vi "GeneralPurposeSOS.vi"() -> ()   [LabVIEW 2015]
uses:
  <userlib>/atmcd32d.llb/EMGainMode_mode typedef.ctl
  <userlib>/atmcd32d.llb/ReadMode_mode typedef.ctl
  <userlib>/atmcd32d.llb/TriggerMode_mode typedef.ctl
  <userlib>/atmcd32d.llb/AcquisitionMode_mode typedef.ctl
  <userlib>/atmcd32d.llb/Shutter_type typedef.ctl
  <userlib>/atmcd32d.llb/Shutter_mode typedef.ctl
  <userlib>/atmcd32d.llb/Spool_method typedef.ctl
  <userlib>/atmcd32d.llb/Tiff_type typedef.ctl
  <vilib>/vision/NI_Vision_Development_Module.lvlib
  <userlib>/libtiff3.llb/libtiff3.lvlib
panel:
  in  "Cooling On":bool
  out "Current Frame 2":i32
  out "Cooling 2":bool
  out "Current T(°C) 2":i32
  in  "Camera Selection":T1(tab)
  in  "Exposure Time(s)":sgl min=0 step=0.1 format="%.2f"
  in  "Camera T(°C)":i32 min=-80 step=1
  in  "Camera DAQ Mode":T2(ring)=enum."Kinetics Series Scan"
  in  "Number of Frames to Acquire":i32 min=0 step=1
  in  "Exposure Time(s) 2":sgl min=0 step=0.1 format="%.2f"
  in  "Camera T(°C)  2":i32 min=-60 step=1
  in  "Camera DAQ Mode 2":T2(ring)=enum."Kinetics Series Scan"
  in  "Number of Frames to Acquire 2":i32 min=0 step=1
  in  "Illumination Mode":enum16{"TIRF", "Dark-Field"}(ring)
  in  "Flip Mirror 2":refnum<k7>(container)
  in  "Save Button":bool
  out "Camera On 2":bool
  out "Current Traj#":u32
  in  "Quit Program":bool
  out "Current Frame":i32
  in  "Start":bool
  in  "Stop":bool
  out "Cooling":bool
  out "Ready":bool
  out "Spot Index":i32
  out "Spot Center":cluster{"X":sgl, "Y":sgl}
  in  "Trajectory Length (s)":dbl=5.0 min=0.0 step=1.0 format="%#_13g"
  in  "Spot Choosing Region":enum16{"Donor", "Acceptor", "Entire Image"}(ring)
  in  "Flip Mirror 1":refnum<k7>(container)
  out "Image View":T3(tab)
  out "Image 3":T4(plugin-control)
  out "Image":T4(plugin-control)
  out "Trajectory":cluster{i32, i32}(graph)
  in  "Terminate Trajectory":bool
  out "error out":errorcluster
  out "Image 2":T4(plugin-control)
  in  "Number of Traj to Acquire":u32 step=1
  in  "Detection Mode":T5(ring)
  in  "Data Saving Path":path
  in  "Experiment Name":string
  out "Camera On":bool
  in  "System Shut Down":bool
  out "Current T(°C)":i32
  # "General-Purpose Single-Object Spectroscopy"
  # "System Settings"
  # "Wide-Field Camera Status"
  # "Spectrograph Status"
  # "Camera Settings"
  # "TIRF-Confocal Settings"
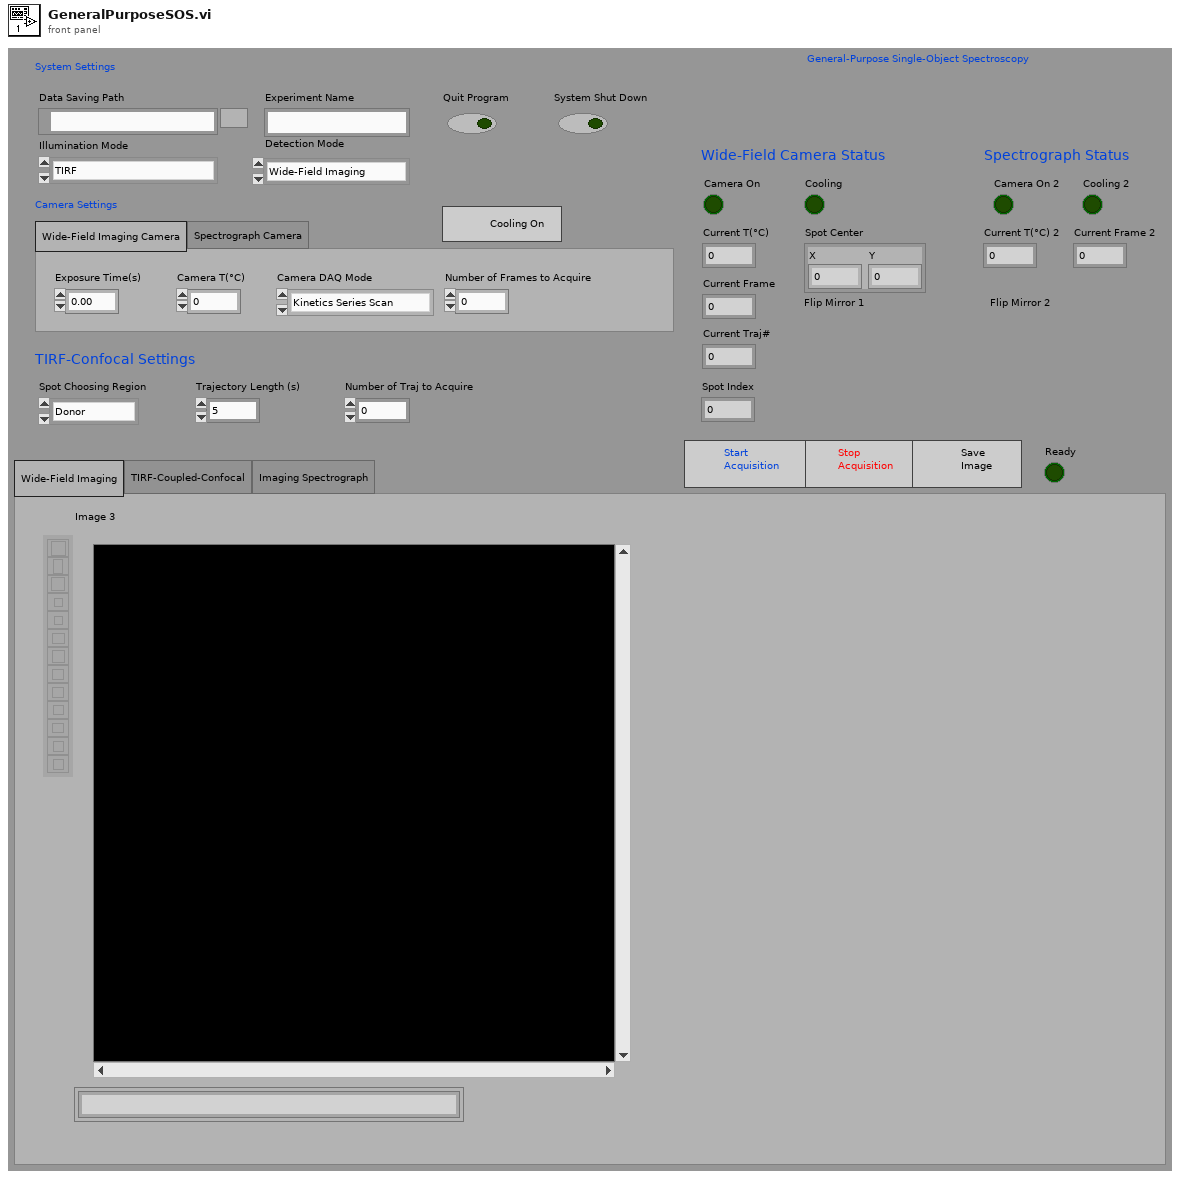
[diagram p1: front panel]
types:
  T1 = enum32{"Wide-Field Imaging Camera", "Spectrograph Camera"}
  T2 = enum16{"Live Monitoring", "Kinetics Series Scan"}
  T3 = enum32{"Wide-Field Imaging", "TIRF-Coupled-Confocal", "Imaging Spectrograph"}
  T4 = typedef "IMAQ Image.ctl" = refnum<image>
  T5 = enum16{"Wide-Field Imaging", "TIRF-Coupled-Confocal", "Imaging Spectrograph"}
  T6 = typedef "AcquisitionMode_mode typedef.ctl" = enum16{"Reserved (0)", "Single Scan", "Accumulate", "Kinetics", "Fast Kinetics", "Run Till Abort", "Reserved (6)", "Reserved (7)", "Reserved (8)", "Time Delayed Integration"}
  T7 = typedef "TriggerMode_mode typedef.ctl" = enum16{"Internal", "External", "N/A (2)", "N/A (3)", "N/A (4)", "N/A (5)", "External Start", "External Exposure (Bulb)", "N/A (8)", "External FVB EM", "Software", "N/A (11)", "External Charge Shifting"}
  T8 = typedef "ReadMode_mode typedef.ctl" = enum16{"Full Vertical Binning", "Multi-Track", "Random-Track", "Single-Track", "Image"}
  T9 = typedef "EMGainMode_mode typedef.ctl" = enum16{"8-bit", "12-bit", "Linear", "Real"}
  T10 = typedef "Shutter_mode typedef.ctl" = enum16{"Auto", "Open", "Close", "N/A (3)", "Open FVB Series", "Open Any Series"}
  T11 = typedef "Shutter_type typedef.ctl" = enum16{"TTL Low", "TTL High"}
  T12 = enum8{"Enabled", "Disabled", "Disabled and Grayed Out"}
  T13 = typedef "Spool_method typedef.ctl" = enum16{"32-bit", "Depends", "16-bit", "Multiple Directory", "Spool to RAM disk", "16-bit FITS", "SIF", "16-buit TIFF", "Multiple Directory Compressed"}
  T14 = typedef "IMAQ Rectangle" = cluster{"Left":i32, "Top":i32, "Right":i32, "Bottom":i32, "Rotation":dbl}
  T15 = typedef "Tiff_type typedef.ctl" = enum16{"8-bit", "16-bit", "color"}
  T16 = typedef "Error Code Enum typedef.ctl" = enum32{"N/A (0)", "DRV_ERROR_CODES", "DRV_SUCCESS", "DRV_VXDNOTINSTALLED", "DRV_ERROR_SCAN", "DRV_ERROR_CHECK_SUM", "DRV_ERROR_FILELOAD", "DRV_UNKNOWN_FUNC", "DRV_ERROR_VXD_INIT", "DRV_ERROR_ADDRESS", "DRV_ERROR_PAGELOCK", "DRV_ERROR_PAGEUNLOCK", "DRV_ERROR_BOARDTEST", "DRV_ERROR_ACK", "DRV_ERROR_UP_FIFO", "DRV_ERROR_PATTERN", "N/A (16)", "DRV_ACQUISITION_ERRORS", "DRV_ACQ_BUFFER", "DRV_ACQ_DOWNFIFO_FULL", "DRV_PROC_UNKONWN_INSTRUCTION", "DRV_ILLEGAL_OP_CODE", "DRV_KINETIC_TIME_NOT_MET", "DRV_ACCUM_TIME_NOT_MET", "DRV_NO_NEW_DATA", "N/A (25)", "DRV_SPOOLERROR", "N/A (27)", "N/A (28)", "N/A (29)", "N/A (30)", "N/A (31)", "N/A (32)", "DRV_TEMPERATURE_CODES", "DRV_TEMPERATURE_OFF", "DRV_TEMPERATURE_NOT_STABILIZED", "DRV_TEMPERATURE_STABILIZED", "DRV_TEMPERATURE_NOT_REACHED", "DRV_TEMPERATURE_OUT_RANGE", "DRV_TEMPERATURE_NOT_SUPPORTED", "DRV_TEMPERATURE_DRIFT", "N/A (41)", "N/A (42)", "N/A (43)", "N/A (44)", "N/A (45)", "N/A (46)", "N/A (47)", "N/A (48)", "DRV_GENERAL_ERRORS", "DRV_INVALID_AUX", "DRV_COF_NOTLOADED", "DRV_FPGAPROG", "DRV_FLEXERROR", "DRV_GPIBERROR", "N/A (55)", "N/A (56)", "N/A (57)", "N/A (58)", "N/A (59)", "N/A (60)", "N/A (61)", "N/A (62)", "N/A (63)", "DRV_DATATYPE", "DRV_DRIVER_ERRORS", "DRV_P1INVALID", "DRV_P2INVALID", "DRV_P3INVALID", "DRV_P4INVALID", "DRV_INIERROR", "DRV_COFERROR", "DRV_ACQUIRING", "DRV_IDLE", "DRV_TEMPCYCLE", "DRV_NOT_INITIALIZED", "DRV_P5INVALID", "DRV_P6INVALID", "DRV_INVALID_MODE", "DRV_INVALID_FILTER", "DRV_I2CERRORS", "DRV_I2CDEVNOTFOUND", "DRV_I2CTIMEOUT", "DRV_P7INVALID", "N/A (84)", "N/A (85)", "N/A (86)", "N/A (87)", "N/A (88)", "N/A (89)", "DRV_IOCERROR", "DRV_VRMVERSIONERROR"}
  T17 = typedef "Image Type" = u32
  T18 = cluster{"Objects":u16, "Threshold":i32, "Reject Border":bool, "Fill Holes":bool, "Min Object Size":bool, "Min Size":i32, "Max Object Size":bool, "Max Size":i32, "Show Search Area":bool, "Show Center":bool, "Show Bounding Box":bool}
  T19 = cluster{"Mean Intensity":sgl, "Standard  Deviation":sgl, "Minimum Intensity":sgl, "Maximum Intensity":sgl}
  T20 = cluster{"Object Center":cluster{"X":sgl, "Y":sgl}, "Bounding Box":cluster{"X Left":i32, "Y Top":i32, "X Right":i32, "Y Bottom":i32}, "Area":sgl, "Orientation":sgl, "Aspect Ratio":sgl, "Nb Holes":i32}[]
  T21 = cluster{"Nb pts X":u32, "Nb pts Y":u32, "xmin":dbl, "xmax":dbl, "ymin":dbl, "ymax":dbl}
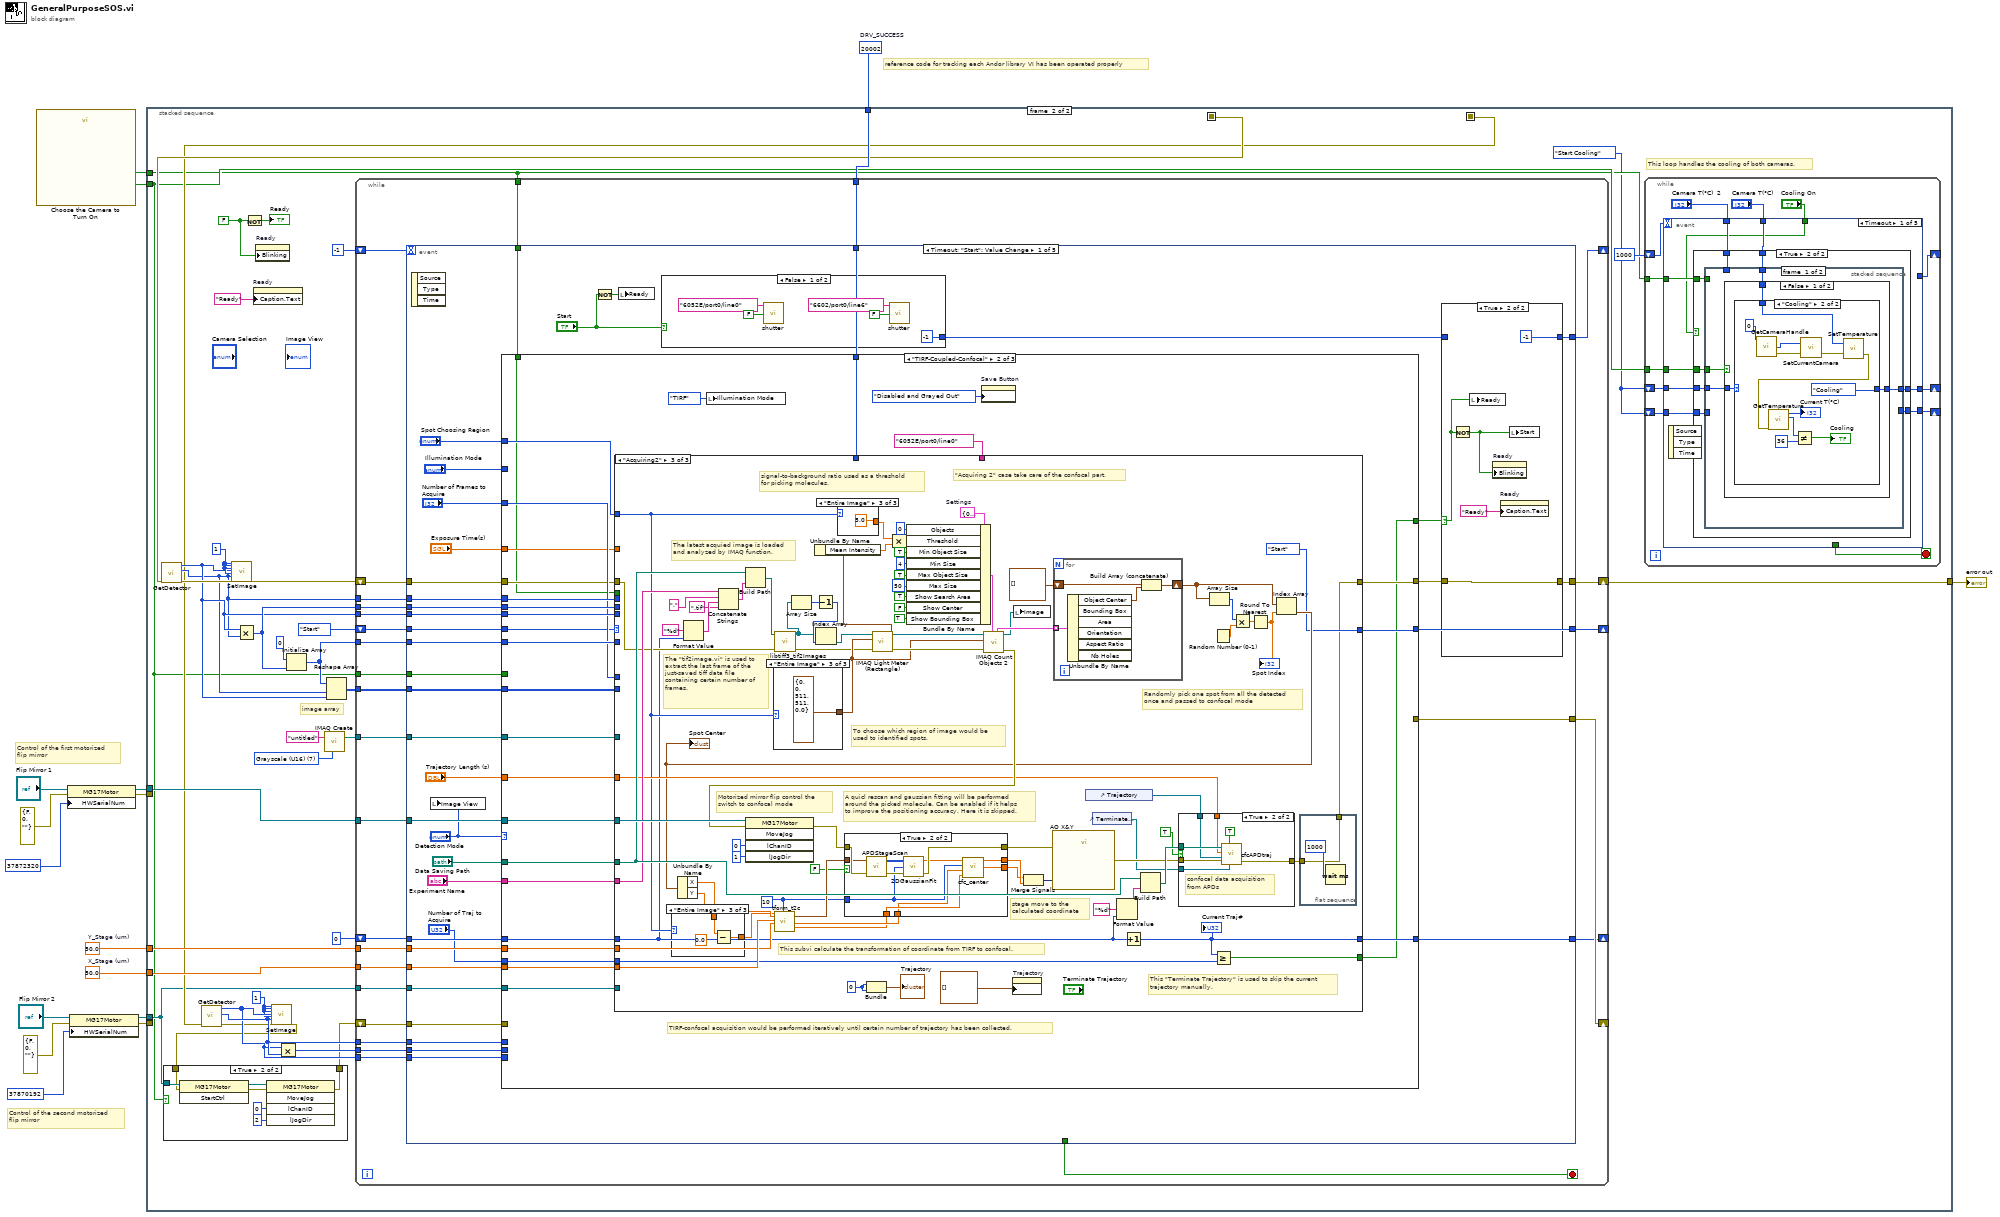
[diagram p0: block diagram]
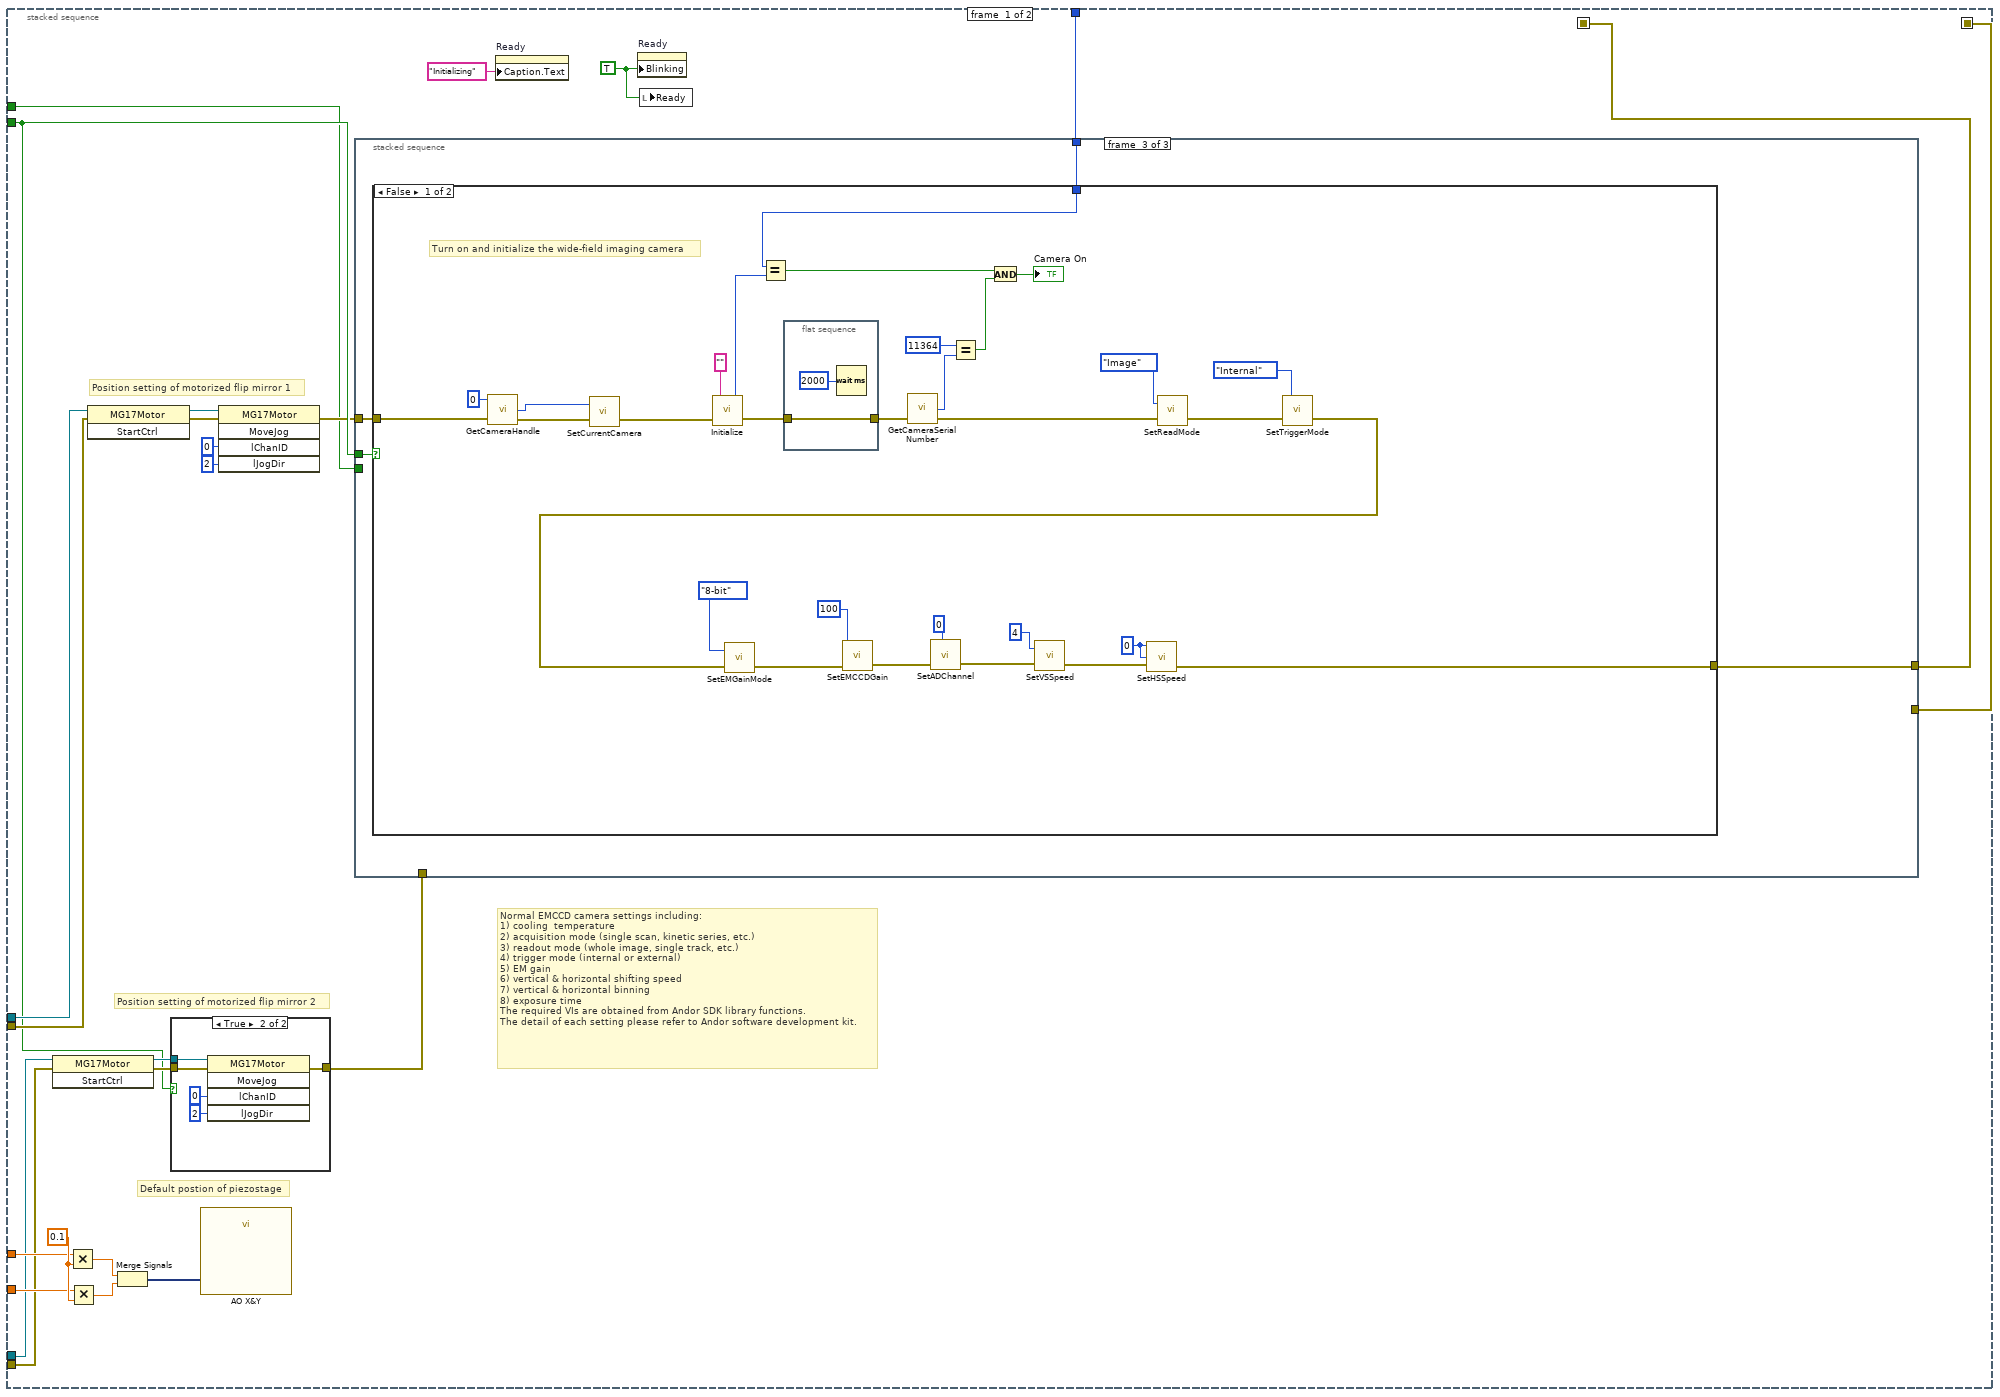
[diagram p2: hidden frame]
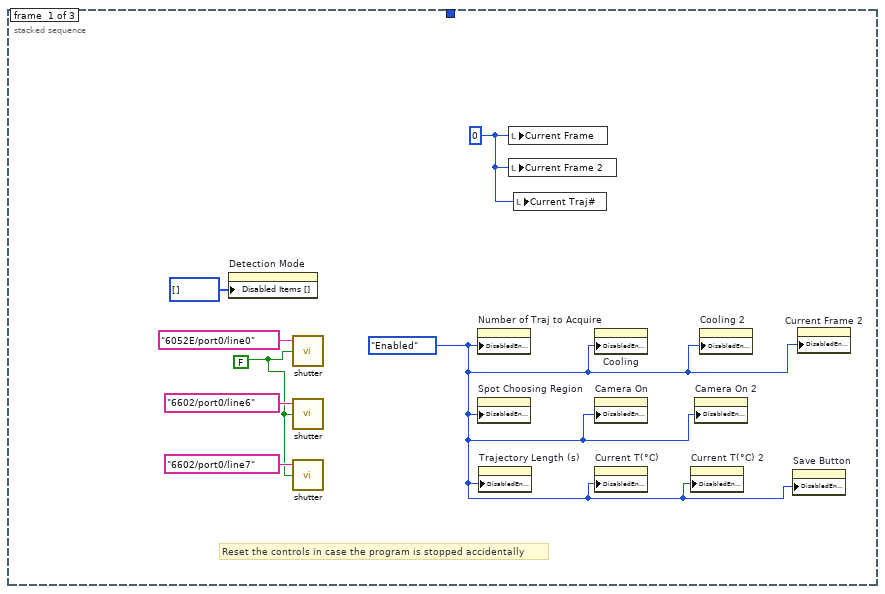
[diagram p3: hidden frame]
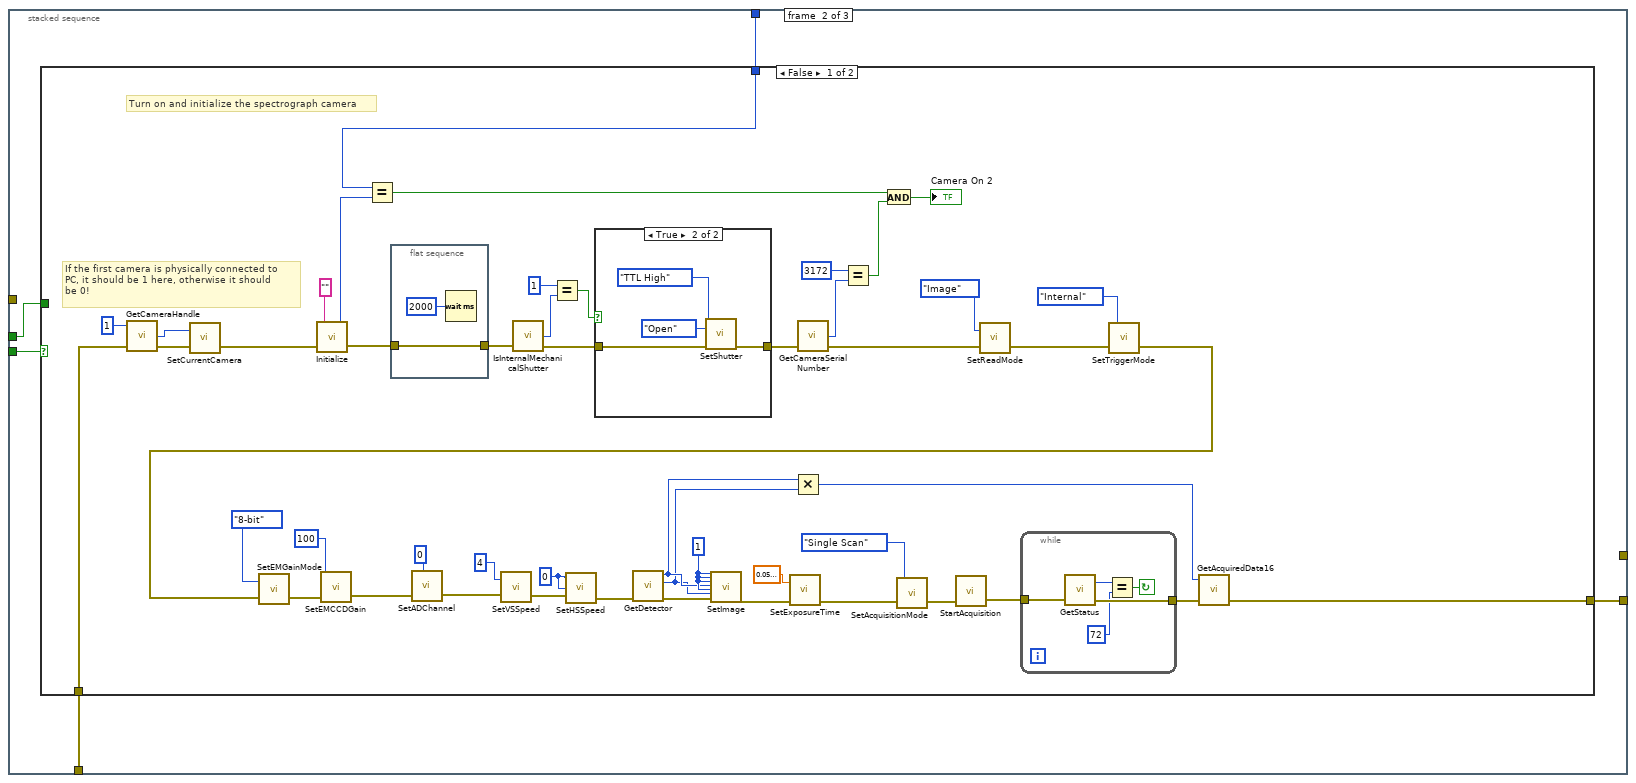
[diagram p4: hidden frame]
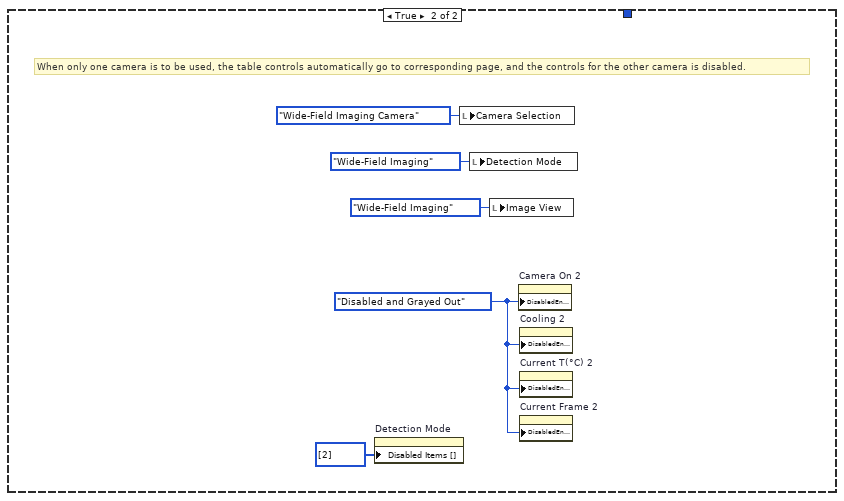
[diagram p6: hidden frame]
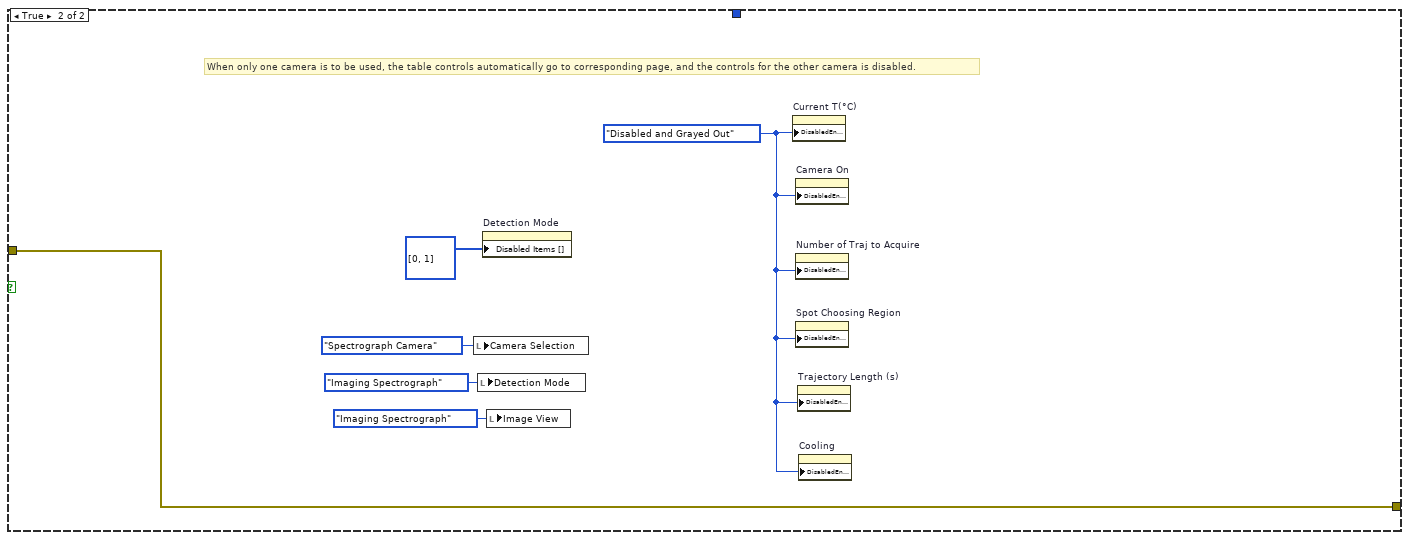
[diagram p7: hidden frame]
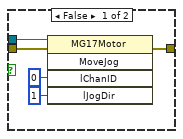
[diagram p8: hidden frame]
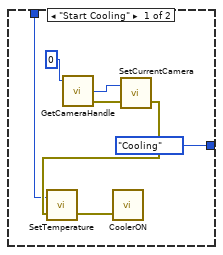
[diagram p10: hidden frame]
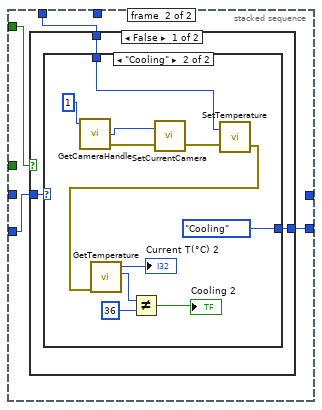
[diagram p12: hidden frame]
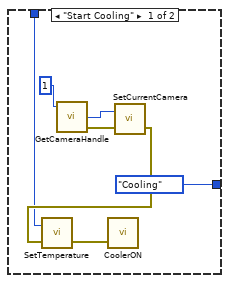
[diagram p13: hidden frame]
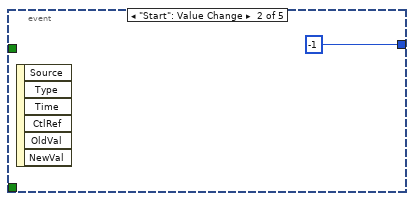
[diagram p15: hidden frame]
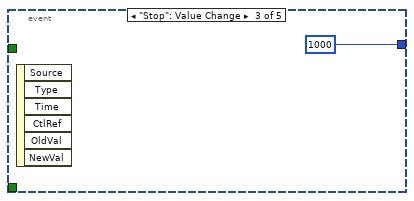
[diagram p16: hidden frame]
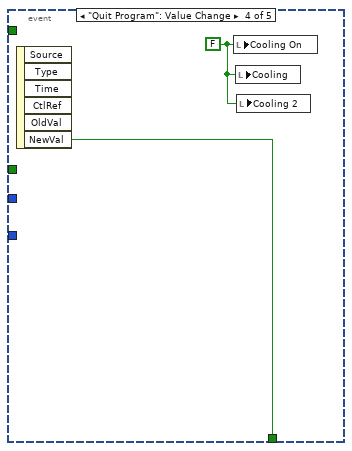
[diagram p17: hidden frame]
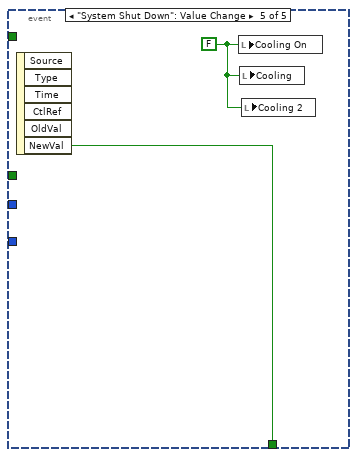
[diagram p18: hidden frame]
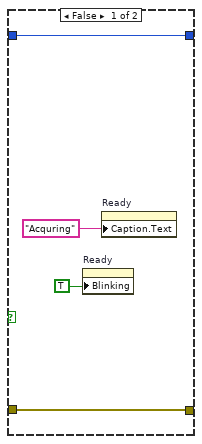
[diagram p20: hidden frame]
diagram:
  w9 = 50.0  # X_Stage (um)
  w10 = 50.0  # Y_Stage (um)
  w16 = 20002  # DRV_SUCCESS
  # "Control of the second motorized \nflip mirror"
  # "Control of the first motorized \nflip mirror"
  # "reference code for tracking each Andor library VI has been operated properly"
  n1 = call "Choose the Camera to Turn On"() -> ("Use spectrograpah camera"=w6:bool, "User wide-field camera"=w7:bool)  [unwired: 16 in, 2 out]
  n2 = property class="MG17Motor"(reference="Flip Mirror 1", error in=errorcluster {"status"=FALSE, "code"=0, "source"=""} ("error in (no error)"), "HWSerialNum"=37872320) -> (reference out=w12:refnum<k7>, error out=w11:errorcluster)
  n3 = property class="MG17Motor"(reference="Flip Mirror 2", error in=errorcluster {"status"=FALSE, "code"=0, "source"=""} ("error in (no error)"), "HWSerialNum"=37870192) -> (reference out=w2:refnum<k7>, error out=w1:errorcluster)
  n4 = stacked-sequence {
    seq-local: [w28 _] -> [_ w189]
    seq-local: [w19 _] -> [_ w185]
    tunnel: w16 -> [w41 w196]
    tunnel: w12 -> [w36 w199]
    tunnel: w11 -> [w35 _]
    tunnel: w10 -> [w32 w197]
    tunnel: w9 -> [w31 w198]
    tunnel: [_ w194] -> w8
    tunnel: w7 -> [w21 w176]
    tunnel: w6 -> [w23 w177]
    tunnel: w2 -> [w25 w182]
    tunnel: w1 -> [w24 _]
    frame #0 {
      w17 = TRUE ("Blinking")
      w33 = 0.1
      # "Position setting of motorized flip mirror 2"
      # "Normal EMCCD camera settings including:\n1) cooling  temperature\n2) acquisition mode (single scan, kinetic series, etc.)\n3) readout mode (whole image, single track, etc.)\n4) trigger mode (internal or external)\n5) EM gain \n6) vertical & horizontal shifting speed\n7) vertical & horizontal binning\n8) exposure time\nThe required VIs are obtained from Andor SDK library functions. \nThe detail of each setting please refer to Andor software development kit."
      # "Position setting of motorized flip mirror 1"
      # "Default postion of piezostage"
      n5 = invoke class="MG17Motor" method="StartCtrl"(reference=w25, error in=w24) -> (reference out=w27:refnum<k7>, error out=w26:errorcluster)  [unwired: 1 in, 1 out]
      n6 = Multiply(x=w32, y=w33) -> (x*y=w30:dbl)
      n7 = Multiply(x=w31, y=w33) -> (x*y=w29:dbl)
      n8 = invoke class="MG17Motor" method="StartCtrl"(reference=w36, error in=w35) -> (reference out=w40:refnum<k7>, error out=w39:errorcluster)  [unwired: 1 in, 1 out]
      n9 = Merge Signals(w30, w29) -> (w34:dynamicdata)
      n10 = case shown="True" w23 {
        tunnel: w27 -> [w163 w170]
        tunnel: w26 -> [w162 w169]
        tunnel: [w161 w166] -> w20
        frame False {
          n11 = invoke class="MG17Motor" method="MoveJog"(reference=w163, error in=w162, "lChanID"=0, "lJogDir"=1) -> (error out=w161:errorcluster)  [unwired: 1 in, 4 out]
        }
        frame True {
          n12 = invoke class="MG17Motor" method="MoveJog"(reference=w170, error in=w169, "lChanID"=0, "lJogDir"=2) -> (error out=w166:errorcluster)  [unwired: 1 in, 4 out]
        }
      }
      n13 = call "AO X&Y"("data"=w34) -> ()  [unwired: 17 in, 2 out]
      n14 = invoke class="MG17Motor" method="MoveJog"(reference=w40, error in=w39, "lChanID"=0, "lJogDir"=2) -> (error out=w22:errorcluster)  [unwired: 1 in, 4 out]
      n15 = stacked-sequence {
        tunnel: w41 -> [_ w51 w122]
        tunnel: w23 -> [_ w49 w121]
        tunnel: w22 -> [_ _ w120]
        tunnel: [_ _ w119] -> w28
        tunnel: w21 -> [_ w53 _]
        tunnel: w20 -> [_ w52 _]
        tunnel: [_ w50 _] -> w19
        frame #0 {
          w43 = 0
          w44 = FALSE
          w42 = T12."Enabled" ("Disabled")
          # "Reset the controls in case the program is stopped accidentally"
          n16 = property on="Detection Mode" class="Enum (strict)"("Disabled Items []"=i32[] []) -> ()  [unwired: 2 in, 2 out]
          n17 = call "shutter.vi"("Boolean"=w44, "lines"=tag "6052E/port0/line0") -> ()  [unwired: 2 in, 1 out]
          n18 = call "shutter.vi"("Boolean"=w44, "lines"=tag "6602/port0/line6") -> ()  [unwired: 2 in, 1 out]
          n19 = call "shutter.vi"("Boolean"=w44, "lines"=tag "6602/port0/line7") -> ()  [unwired: 2 in, 1 out]
          n20 = property on="Number of Traj to Acquire" class="DigNum (strict)"("DisabledEnum"=w42) -> ()  [unwired: 2 in, 2 out]
          n21 = property on="Spot Choosing Region" class="Enum (strict)"("DisabledEnum"=w42) -> ()  [unwired: 2 in, 2 out]
          n22 = property on="Trajectory Length (s)" class="DigNum (strict)"("DisabledEnum"=w42) -> ()  [unwired: 2 in, 2 out]
          n23 = local write "Current Frame"(w43) -> ()
          n24 = local write "Current Frame 2"(w43) -> ()
          n25 = local write "Current Traj#"(w43) -> ()
          n26 = property on="Cooling" class="Bool (strict)"("DisabledEnum"=w42) -> ()  [unwired: 2 in, 2 out]
          n27 = property on="Camera On" class="Bool (strict)"("DisabledEnum"=w42) -> ()  [unwired: 2 in, 2 out]
          n28 = property on="Current T(°C)" class="DigNum (strict)"("DisabledEnum"=w42) -> ()  [unwired: 2 in, 2 out]
          n29 = property on="Current T(°C) 2" class="DigNum (strict)"("DisabledEnum"=w42) -> ()  [unwired: 2 in, 2 out]
          n30 = property on="Camera On 2" class="Bool (strict)"("DisabledEnum"=w42) -> ()  [unwired: 2 in, 2 out]
          n31 = property on="Cooling 2" class="Bool (strict)"("DisabledEnum"=w42) -> ()  [unwired: 2 in, 2 out]
          n32 = property on="Save Button" class="Bool"("DisabledEnum"=w42) -> ()  [unwired: 2 in, 2 out]
          n33 = property on="Current Frame 2" class="DigNum (strict)"("DisabledEnum"=w42) -> ()  [unwired: 2 in, 2 out]
        }
        frame #1 {
          n34 = case shown="False" w53 {
            tunnel: [w62 _] -> w50
            tunnel: w52 -> [w70 _]
            tunnel: w51 -> [w69 _]
            tunnel: w49 -> [_ _]
            frame False {
              w59 = 1
              w87 = 0
              # "Turn on and initialize the spectrograph camera"
              # "If the first camera is physically connected to \nPC, it should be 1 here, otherwise it should \nbe 0!"
              n35 = call <userlib>:"GetCameraHandle.vi"("error in (no error)"=w70, "cameraIndex"=1) -> ("error out"=w85:errorcluster, "cameraHandle"=w83:i32)  [unwired: 1 in, 1 out]
              n36 = call <userlib>:"SetCurrentCamera.vi"("error in (no error)"=w85, "cameraHandle"=w83) -> ("error out"=w84:errorcluster)  [unwired: 1 out]
              n37 = call <userlib>:"Initialize.vi"("error in (no error)"=w84, "directory (\"\")"="") -> ("error out"=w99:errorcluster, "DLL error code"=w100:u32)
              n38 = Equal?(x=w69, y=w100) -> (x = y?=w75:bool)
              n39 = flat-sequence {
                tunnel: w99 -> [w112]
                tunnel: [w112] -> w78
                frame #0 {
                  n40 = Wait (ms)(milliseconds to wait=u32 2000) -> ()  [unwired: 1 out]
                }
              }
              n41 = call <userlib>:"IsInternalMechanicalShutter.vi"("error in (no error)"=w78) -> ("error out"=w77:errorcluster, "InternalShutter"=w72:i32)  [unwired: 2 in, 1 out]
              n42 = Equal?(x=1, y=w72) -> (x = y?=w73:bool)
              n43 = case shown="True" w73 {
                tunnel: w77 -> [w107 w111]
                tunnel: [w107 w110] -> w76
                frame False {
                }
                frame True {
                  n44 = call <userlib>:"SetShutter.vi"("type"=Shutter_type_typedef."TTL High", "mode"=Shutter_mode_typedef."Open", "error in (no error)"=w111) -> ("error out"=w110:errorcluster)  [unwired: 11 in, 1 out]
                }
              }
              n45 = call <userlib>:"GetCameraSerialNumber.vi"("error in (no error)"=w76) -> ("error out"=w61:errorcluster, "number"=w81:i32)  [unwired: 2 in, 1 out]
              n46 = Equal?(x=3172, y=w81) -> (x = y?=w79:bool)
              n47 = And(x=w75, y=w79) -> (x .and. y?=→"Camera On 2":bool)
              n48 = call <userlib>:"SetReadMode.vi"("error in (no error)"=w61, "mode"=ReadMode_mode_typedef."Image" ("Read Mode")) -> ("error out"=w96:errorcluster)  [unwired: 1 out]
              n49 = call <userlib>:"SetTriggerMode.vi"("error in (no error)"=w96, "mode"=TriggerMode_mode_typedef."Internal" ("Trigger Mode")) -> ("error out"=w88:errorcluster)  [unwired: 1 out]
              n50 = call <userlib>:"SetEMGainMode.vi"("error in (no error)"=w88, "mode"=EMGainMode_mode_typedef."8-bit") -> ("error out"=w89:errorcluster)  [unwired: 1 out]
              n51 = call <userlib>:"SetEMCCDGain.vi"("error in (no error)"=w89, "gain"=100 ("EM Gain")) -> ("error out"=w91:errorcluster)  [unwired: 1 out]
              n52 = call <userlib>:"SetADChannel.vi"("error in (no error)"=w91, "channel"=0) -> ("error out"=w93:errorcluster)  [unwired: 1 out]
              n53 = call <userlib>:"SetVSSpeed.vi"("error in (no error)"=w93, "index"=4) -> ("error out"=w92:errorcluster)  [unwired: 1 out]
              n54 = call <userlib>:"SetHSSpeed.vi"("error in (no error)"=w92, "index"=w87, "type"=w87) -> ("error out"=w58:errorcluster)  [unwired: 1 in, 1 out]
              n55 = call <userlib>:"GetDetector.vi"("error in (no error)"=w58) -> ("error out"=w57:errorcluster, "ypixels"=w55:i32, "xpixels"=w56:i32)  [unwired: 3 in, 1 out]
              n56 = call <userlib>:"SetImage.vi"("hbin"=w59, "vbin"=w59, "hstart"=w59, "hend"=w56, "vstart"=w59, "vend"=w55, "error in (no error)"=w57) -> ("error out"=w60:errorcluster)  [unwired: 19 in, 1 out]
              n57 = call <userlib>:"SetExposureTime.vi"("error in (no error)"=w60, "time"=sgl 0.05) -> ("error out"=w66:errorcluster)  [unwired: 1 out]
              n58 = Multiply(x=w56, y=w55) -> (x*y=w54:i32)
              n59 = call <userlib>:"SetAcquisitionMode.vi"("error in (no error)"=w66, "mode"=AcquisitionMode_mode_typedef."Single Scan") -> ("error out"=w65:errorcluster)  [unwired: 1 out]
              n60 = call <userlib>:"StartAcquisition.vi"("error in (no error)"=w65) -> ("error out"=w64:errorcluster)  [unwired: 1 in, 1 out]
              n61 = while {
                tunnel: w64 -> [w106]
                tunnel: [w105] -> w63
                stop <- w104 continue-if-true
                n62 = call <userlib>:"GetStatus.vi"("error in (no error)"=w106) -> ("error out"=w105:errorcluster, "status"=w103:T16)  [unwired: 2 in, 1 out]
                n63 = Equal?(x=w103, y=72) -> (x = y?=w104:bool)
              }
              n64 = call <userlib>:"GetAcquiredData16.vi"("error in (no error)"=w63, "size"=w54) -> ("error out"=w62:errorcluster)  [unwired: 1 in, 2 out]
            }
            frame True {
              w115 = T12."Disabled and Grayed Out" ("Disabled")
              # "When only one camera is to be used, the table controls automatically go to corresponding page, and the controls for the other camera is disabled."
              n65 = property on="Detection Mode" class="Enum (strict)"("Disabled Items []"=i32[] [2]) -> ()  [unwired: 2 in, 2 out]
              n66 = local write "Camera Selection"(T1."Wide-Field Imaging Camera" ("Camera Selection")) -> ()
              n67 = local write "Detection Mode"(T5."Wide-Field Imaging" ("Detection Mode")) -> ()
              n68 = local write "Image View"(T3."Wide-Field Imaging" ("Image View")) -> ()
              n69 = property on="Camera On 2" class="Bool (strict)"("DisabledEnum"=w115) -> ()  [unwired: 2 in, 2 out]
              n70 = property on="Cooling 2" class="Bool (strict)"("DisabledEnum"=w115) -> ()  [unwired: 2 in, 2 out]
              n71 = property on="Current T(°C) 2" class="DigNum (strict)"("DisabledEnum"=w115) -> ()  [unwired: 2 in, 2 out]
              n72 = property on="Current Frame 2" class="DigNum (strict)"("DisabledEnum"=w115) -> ()  [unwired: 2 in, 2 out]
            }
          }
        }
        frame #2 {
          n73 = case shown="False" w121 {
            tunnel: w122 -> [w152 _]
            tunnel: w120 -> [w134 w159]
            tunnel: [w124 w159] -> w119
            frame False {
              w137 = 0
              # "Turn on and initialize the wide-field imaging camera"
              n74 = call <userlib>:"GetCameraHandle.vi"("error in (no error)"=w134, "cameraIndex"=0) -> ("error out"=w135:errorcluster, "cameraHandle"=w132:i32)  [unwired: 1 in, 1 out]
              n75 = call <userlib>:"SetCurrentCamera.vi"("error in (no error)"=w135, "cameraHandle"=w132) -> ("error out"=w133:errorcluster)  [unwired: 1 out]
              n76 = call <userlib>:"Initialize.vi"("error in (no error)"=w133, "directory (\"\")"="") -> ("error out"=w149:errorcluster, "DLL error code"=w150:u32)
              n77 = Equal?(x=w152, y=w150) -> (x = y?=w127:bool)
              n78 = flat-sequence {
                tunnel: w149 -> [w153]
                tunnel: [w153] -> w130
                frame #0 {
                  n79 = Wait (ms)(milliseconds to wait=u32 2000) -> ()  [unwired: 1 out]
                }
              }
              n80 = call <userlib>:"GetCameraSerialNumber.vi"("error in (no error)"=w130) -> ("error out"=w123:errorcluster, "number"=w129:i32)  [unwired: 2 in, 1 out]
              n81 = Equal?(x=11364, y=w129) -> (x = y?=w125:bool)
              n82 = And(x=w127, y=w125) -> (x .and. y?=→"Camera On":bool)
              n83 = call <userlib>:"SetReadMode.vi"("error in (no error)"=w123, "mode"=ReadMode_mode_typedef."Image" ("Read Mode")) -> ("error out"=w146:errorcluster)  [unwired: 1 out]
              n84 = call <userlib>:"SetTriggerMode.vi"("error in (no error)"=w146, "mode"=TriggerMode_mode_typedef."Internal" ("Trigger Mode")) -> ("error out"=w138:errorcluster)  [unwired: 1 out]
              n85 = call <userlib>:"SetEMGainMode.vi"("error in (no error)"=w138, "mode"=EMGainMode_mode_typedef."8-bit") -> ("error out"=w139:errorcluster)  [unwired: 1 out]
              n86 = call <userlib>:"SetEMCCDGain.vi"("error in (no error)"=w139, "gain"=100 ("EM Gain")) -> ("error out"=w141:errorcluster)  [unwired: 1 out]
              n87 = call <userlib>:"SetADChannel.vi"("error in (no error)"=w141, "channel"=0) -> ("error out"=w143:errorcluster)  [unwired: 1 out]
              n88 = call <userlib>:"SetVSSpeed.vi"("error in (no error)"=w143, "index"=4) -> ("error out"=w142:errorcluster)  [unwired: 1 out]
              n89 = call <userlib>:"SetHSSpeed.vi"("error in (no error)"=w142, "index"=w137, "type"=w137) -> ("error out"=w124:errorcluster)  [unwired: 1 in, 1 out]
            }
            frame True {
              w158 = T12."Disabled and Grayed Out" ("Disabled")
              # "When only one camera is to be used, the table controls automatically go to corresponding page, and the controls for the other camera is disabled."
              n90 = local write "Camera Selection"(T1."Spectrograph Camera" ("Tab Control")) -> ()
              n91 = local write "Detection Mode"(T5."Imaging Spectrograph" ("Detection Mode")) -> ()
              n92 = property on="Detection Mode" class="Enum (strict)"("Disabled Items []"=i32[] [0, 1]) -> ()  [unwired: 2 in, 2 out]
              n93 = local write "Image View"(T3."Imaging Spectrograph" ("Image View")) -> ()
              n94 = property on="Current T(°C)" class="DigNum (strict)"("DisabledEnum"=w158) -> ()  [unwired: 2 in, 2 out]
              n95 = property on="Camera On" class="Bool (strict)"("DisabledEnum"=w158) -> ()  [unwired: 2 in, 2 out]
              n96 = property on="Number of Traj to Acquire" class="DigNum (strict)"("DisabledEnum"=w158) -> ()  [unwired: 2 in, 2 out]
              n97 = property on="Spot Choosing Region" class="Enum (strict)"("DisabledEnum"=w158) -> ()  [unwired: 2 in, 2 out]
              n98 = property on="Trajectory Length (s)" class="DigNum (strict)"("DisabledEnum"=w158) -> ()  [unwired: 2 in, 2 out]
              n99 = property on="Cooling" class="Bool (strict)"("DisabledEnum"=w158) -> ()  [unwired: 2 in, 2 out]
            }
          }
        }
      }
      n100 = property on="Ready" class="Bool (strict)"("Caption.Text"="Initializing") -> ()  [unwired: 2 in, 2 out]
      n101 = property on="Ready" class="Bool (strict)"("Blinking"=w17) -> ()  [unwired: 2 in, 2 out]
      n102 = local write "Ready"(w17) -> ()
    }
    frame #1 {
      w174 = 1
      w175 = enum16{"Start Cooling", "Cooling"}."Start Cooling"
      w192 = T17 7 items=["Grayscale (U8)", "Grayscale (I16)", "Grayscale (SGL)", "Complex (CSG)", "RGB (U32)", "HSL (U32)", "RGB (U64)", "Grayscale (U16)"] ("Image Type")
      w171 = FALSE ("Cooling")
      w207 = 1
      # "This loop handles the cooling of both cameras."
      # "image array"
      n103 = call <userlib>:"GetDetector.vi"("error in (no error)"=w189) -> ("error out"=w206:errorcluster, "ypixels"=w200:i32, "xpixels"=w201:i32)  [unwired: 3 in, 1 out]
      n104 = call <userlib>:"GetDetector.vi"("error in (no error)"=w185) -> ("error out"=w173:errorcluster, "ypixels"=w187:i32, "xpixels"=w186:i32)  [unwired: 3 in, 1 out]
      n105 = call <userlib>:"SetImage.vi"("hbin"=w207, "vbin"=w207, "hstart"=w207, "hend"=w201, "vstart"=w207, "vend"=w200, "error in (no error)"=w206) -> ("error out"=w193:errorcluster)  [unwired: 19 in, 1 out]
      n106 = Multiply(x=w201, y=w200) -> (x*y=w202:i32)
      n107 = Not(x=w171) -> (.not. x?=→"Ready":bool)
      n108 = property on="Ready" class="Bool (strict)"("Caption.Text"="Ready") -> ()  [unwired: 2 in, 2 out]
      n109 = property on="Ready" class="Bool (strict)"("Blinking"=w171) -> ()  [unwired: 2 in, 2 out]
      n110 = call <userlib>:"SetImage.vi"("hbin"=w174, "vbin"=w174, "hstart"=w174, "hend"=w186, "vstart"=w174, "vend"=w187, "error in (no error)"=w173) -> ("error out"=w183:errorcluster)  [unwired: 19 in, 1 out]
      n111 = case shown="True" w177 {
        tunnel: [w295 w302] -> w184
        tunnel: w182 -> [_ w301]
        tunnel: w183 -> [w295 w296]
        frame False {
        }
        frame True {
          n112 = invoke class="MG17Motor" method="StartCtrl"(reference=w301, error in=w296) -> (reference out=w300:refnum<k7>, error out=w299:errorcluster)  [unwired: 1 in, 1 out]
          n113 = invoke class="MG17Motor" method="MoveJog"(reference=w300, error in=w299, "lChanID"=0, "lJogDir"=2) -> (error out=w302:errorcluster)  [unwired: 1 in, 4 out]
        }
      }
      n114 = Multiply(x=w186, y=w187) -> (x*y=w188:i32)
      n115 = Initialize Array(0, w202) -> (w203:i32[])
      n116 = call "IMAQ Create"("Image Name"="untitled", "Image Type"=w192) -> ("New Image"=w190:T4)  [unwired: 3 in, 1 out]
      n117 = Reshape Array(w203, w200, w201) -> (w204:i32[][])
      n118 = while {
        tunnel: w204 -> [w329]
        tunnel: w203 -> [w328]
        tunnel: w202 -> [w327]
        tunnel: w201 -> [w326]
        tunnel: w200 -> [w325]
        tunnel: w199 -> [w324]
        tunnel: w198 -> [w323]
        tunnel: w197 -> [w322]
        tunnel: w196 -> [w321]
        shift-right: [w317] -> w194
        shift-left: w193 -> [w315]
        shift-right: [w319] -> _
        shift-left: -1 -> [w320]
        tunnel: w190 -> [w316]
        tunnel: w188 -> [w314]
        tunnel: w187 -> [w313]
        tunnel: w186 -> [w312]
        shift-right: [w310] -> _
        shift-left: w184 -> [w311]
        tunnel: w182 -> [w309]
        tunnel: w177 -> [w308]
        tunnel: w176 -> [w307]
        shift-right: [w306] -> _
        shift-left: u32 0 -> [w303]
        shift-right: [w304] -> _
        shift-left: enum16{"Start", "Acquiring", "Acquiring2"}."Start" -> [w305]
        stop <- w318 stop-if-true
        n119 = event shown="[0] Timeout;  \"Start\": Value Change" {
          selector: _ -> [_ _ _ _ _]
          dyn-events: _ -> [_ _ _ _ _]
          timeout: w320 -> [_ _ _ _ _]
          tunnel: w329 -> [w368 _ _ _ _]
          tunnel: w328 -> [w367 _ _ _ _]
          tunnel: w327 -> [w366 _ _ _ _]
          tunnel: w326 -> [w365 _ _ _ _]
          tunnel: w325 -> [w364 _ _ _ _]
          tunnel: w303 -> [w363 _ _ _ _]
          tunnel: w324 -> [w362 _ _ w995 _]
          tunnel: w323 -> [w361 _ _ _ _]
          tunnel: w322 -> [w360 _ _ _ _]
          tunnel: w321 -> [w359 _ _ w994 _]
          tunnel: [w355 _ _ _ _] -> w317
          tunnel: [w357 -1 -1 _ _] -> w319
          tunnel: [_ _ _ w993 w1074] -> w318
          tunnel: w316 -> [w353 _ _ _ _]
          tunnel: w315 -> [w336 _ _ _ _]
          tunnel: w311 -> [w345 _ _ _ _]
          tunnel: w314 -> [w344 _ _ _ _]
          tunnel: w313 -> [w343 _ _ _ _]
          tunnel: w312 -> [w342 _ _ _ _]
          tunnel: [w341 _ _ _ _] -> w310
          tunnel: w309 -> [w340 _ _ w989 _]
          tunnel: w308 -> [w339 _ _ w986 _]
          tunnel: w307 -> [w338 _ _ w988 _]
          tunnel: [w335 _ _ _ _] -> w306
          tunnel: w305 -> [w334 _ _ _ _]
          tunnel: [w333 _ _ _ _] -> w304
          event Timeout; "Start": Value Change {
            n120 = event-data() -> ()  [unwired: 1 in, 3 out]
            n121 = local write "Image View"("Detection Mode") -> ()
            n122 = case shown="\"TIRF-Coupled-Confocal\"" "Detection Mode" {
              tunnel: w359 -> [w404 w582 w800]
              tunnel: w336 -> [w390 w561 _]
              tunnel: w368 -> [_ w581 _]
              tunnel: w367 -> [w402 w580 w799]
              tunnel: w366 -> [w403 w579 w798]
              tunnel: w365 -> [w401 w578 w796]
              tunnel: w364 -> [w386 w577 w797]
              tunnel: "Data Saving Path" -> [w400 w576 w804]
              tunnel: "Experiment Name" -> [w399 w575 w803]
              tunnel: w363 -> [_ w564 _]
              tunnel: w362 -> [w388 w574 w810]
              tunnel: w361 -> [_ w573 _]
              tunnel: w360 -> [_ w572 _]
              tunnel: "Spot Choosing Region" -> [_ w571 _]
              tunnel: "Trajectory Length (s)" -> [_ w570 _]
              tunnel: [w395 w558 _] -> w356
              tunnel: "Number of Frames to Acquire" -> [w398 w569 _]
              tunnel: [w397 w556 w795] -> w354
              tunnel: "Exposure Time(s)" -> [w393 w568 _]
              tunnel: w353 -> [w394 w560 w807]
              tunnel: w345 -> [_ _ w811]
              tunnel: w344 -> [_ _ w817]
              tunnel: w343 -> [_ _ w816]
              tunnel: w342 -> [_ _ w815]
              tunnel: [_ _ w809] -> w341
              tunnel: w340 -> [w389 w566 w814]
              tunnel: w339 -> [_ _ w794]
              tunnel: w338 -> [w387 w555 _]
              tunnel: "Illumination Mode" -> [w392 _ w813]
              tunnel: [_ w565 _] -> w335
              tunnel: w334 -> [w385 w562 w802]
              tunnel: [w384 w563 w801] -> w333
              tunnel: "Number of Traj to Acquire" -> [_ w557 _]
              frame "Wide-Field Imaging" {
                # "Illumination mode is set by the open/close of \nmotorized shutter in corresponding optical path."
                n123 = case shown="\"TIRF\"" w392 {
                  tunnel: [tag "6052E/port0/line0" ("lines") tag "6602/port0/line6" ("lines")] -> w391
                  frame "TIRF" {
                  }
                  frame "Dark-Field" {
                  }
                }
                n124 = case shown="\"Kinetics Series Scan\"" "Camera DAQ Mode" {
                  tunnel: w404 -> [_ w462]
                  tunnel: w390 -> [w416 w470]
                  tunnel: w403 -> [w409 w467]
                  tunnel: w402 -> [_ w468]
                  tunnel: w386 -> [w439 w465]
                  tunnel: w401 -> [w438 w464]
                  tunnel: w400 -> [_ w472]
                  tunnel: w399 -> [_ w473]
                  tunnel: [w408 w463] -> w395
                  tunnel: w398 -> [_ w475]
                  tunnel: [FALSE w461] -> w397
                  tunnel: w394 -> [w423 w466]
                  tunnel: w393 -> [w410 w457]
                  tunnel: w391 -> [w425 w469]
                  tunnel: w389 -> [w415 w460]
                  tunnel: w388 -> [w414 w459]
                  tunnel: w387 -> [w413 w458]
                  tunnel: w385 -> [_ w456]
                  tunnel: [_ w455] -> w384
                  frame "Live Monitoring" {
                    # "Set the position of the two flip mirror to achieve certain optical path."
                    # "Use \"GetCameraHandle.vi\" + \"SetCurrentCamera.vi\" to \nselect correct camera when dealing with multiple cameras."
                    n125 = case shown="False" w413 {
                      tunnel: w415 -> [w448 _]
                      tunnel: [w444 w449] -> w407
                      tunnel: w416 -> [w447 w449]
                      frame False {
                        n126 = invoke class="MG17Motor" method="MoveJog"(reference=w448, error in=w447, "lChanID"=0, "lJogDir"=1) -> (error out=w444:errorcluster)  [unwired: 1 in, 4 out]
                      }
                      frame True {
                      }
                    }
                    n127 = property on="Save Button" class="Bool"("DisabledEnum"=T12."Enabled" ("Disabled")) -> ()  [unwired: 2 in, 2 out]
                    n128 = invoke class="MG17Motor" method="MoveJog"(reference=w414, error in=w407, "lChanID"=0, "lJogDir"=2) -> (error out=w417:errorcluster)  [unwired: 1 in, 4 out]
                    n129 = call <userlib>:"GetCameraHandle.vi"("error in (no error)"=w417, "cameraIndex"=0) -> ("error out"=w418:errorcluster, "cameraHandle"=w419:i32)  [unwired: 1 in, 1 out]
                    n130 = call <userlib>:"SetCurrentCamera.vi"("error in (no error)"=w418, "cameraHandle"=w419) -> ("error out"=w411:errorcluster)  [unwired: 1 out]
                    n131 = call <userlib>:"SetExposureTime.vi"("error in (no error)"=w411, "time"=w410) -> ("error out"=w412:errorcluster)  [unwired: 1 out]
                    n132 = call <userlib>:"SetAcquisitionMode.vi"("error in (no error)"=w412, "mode"=AcquisitionMode_mode_typedef."Single Scan") -> ("error out"=w436:errorcluster)  [unwired: 1 out]
                    n133 = call <userlib>:"SetSpool.vi"("active"=FALSE, "method"=Spool_method_typedef."16-buit TIFF", "name"="", "error in (no error)"=w436) -> ("error out"=w435:errorcluster)  [unwired: 10 in, 1 out]
                    n134 = call "shutter.vi"("error in (no error)"=w435, "Boolean"=TRUE, "lines"=w425) -> ("error out"=w441:errorcluster)  [unwired: 1 in]
                    n135 = call <userlib>:"StartAcquisition.vi"("error in (no error)"=w441) -> ("error out"=w443:errorcluster)  [unwired: 1 in, 1 out]
                    n136 = while {
                      tunnel: w443 -> [w452]
                      tunnel: [w454] -> w429
                      stop <- w450 continue-if-true
                      n137 = call <userlib>:"GetStatus.vi"("error in (no error)"=w452) -> ("error out"=w454:errorcluster, "status"=w451:T16)  [unwired: 2 in, 1 out]
                      n138 = Equal?(x=w451, y=72) -> (x = y?=w450:bool)
                    }
                    n139 = call <userlib>:"GetAcquiredData16.vi"("error in (no error)"=w429, "size"=w409) -> ("error out"=w408:errorcluster, "array"=w428:u16[])  [unwired: 1 in, 1 out]
                    n140 = Multiply(x=w428, y=1) -> (x*y=w426:i32[])
                    n141 = Reshape Array(w426, w439, w438) -> (w431:i32[][])
                    n142 = call "IMAQ ArrayToImage"("Image Pixels (U16)"=w431, "Image"=w423) -> ("Image Out"=→"Image 3":T4)  [unwired: 8 in, 1 out]
                  }
                  frame "Kinetics Series Scan" {
                    n143 = Build Path(base path=w472, name or relative path=w473) -> (appended path=w474:path)
                    n144 = Path To String(path=w474) -> (string=w471:string)
                    n145 = case shown="\"Start\"" w456 {
                      tunnel: w475 -> [w500 _ _]
                      tunnel: w471 -> [w497 _ _]
                      tunnel: w470 -> [w486 w529 w553]
                      tunnel: w469 -> [w495 w521 _]
                      tunnel: [enum16{"Start", "Acquiring", "Acquiring2"}."Acquiring" w517 _] -> w455
                      tunnel: w468 -> [_ w528 _]
                      tunnel: w467 -> [_ w527 _]
                      tunnel: w466 -> [_ w526 _]
                      tunnel: w465 -> [_ w525 _]
                      tunnel: w464 -> [_ w524 _]
                      tunnel: [w482 w519 w553] -> w463
                      tunnel: w462 -> [_ w523 _]
                      tunnel: [FALSE w518 _] -> w461
                      tunnel: w460 -> [w485 _ _]
                      tunnel: w459 -> [w484 _ _]
                      tunnel: w458 -> [w481 _ _]
                      tunnel: w457 -> [w478 w514 _]
                      frame "Start" {
                        # "\"kinetics\" mode by defalut will save all frames automatically, \nby enabling the SetSpool.vi."
                        # "open shutter"
                        n146 = case shown="False" w481 {
                          tunnel: w485 -> [w510 _]
                          tunnel: [w506 w511] -> w476
                          tunnel: w486 -> [w509 w511]
                          frame False {
                            n147 = invoke class="MG17Motor" method="MoveJog"(reference=w510, error in=w509, "lChanID"=0, "lJogDir"=1) -> (error out=w506:errorcluster)  [unwired: 1 in, 4 out]
                          }
                          frame True {
                          }
                        }
                        n148 = property on="Save Button" class="Bool"("DisabledEnum"=T12."Disabled and Grayed Out" ("Disabled")) -> ()  [unwired: 2 in, 2 out]
                        n149 = invoke class="MG17Motor" method="MoveJog"(reference=w484, error in=w476, "lChanID"=0, "lJogDir"=2) -> (error out=w483:errorcluster)  [unwired: 1 in, 4 out]
                        n150 = call <userlib>:"GetCameraHandle.vi"("error in (no error)"=w483, "cameraIndex"=0) -> ("error out"=w492:errorcluster, "cameraHandle"=w491:i32)  [unwired: 1 in, 1 out]
                        n151 = call <userlib>:"SetCurrentCamera.vi"("error in (no error)"=w492, "cameraHandle"=w491) -> ("error out"=w489:errorcluster)  [unwired: 1 out]
                        n152 = call <userlib>:"SetAcquisitionMode.vi"("error in (no error)"=w489, "mode"=AcquisitionMode_mode_typedef."Kinetics") -> ("error out"=w479:errorcluster)  [unwired: 1 out]
                        n153 = call <userlib>:"SetExposureTime.vi"("error in (no error)"=w479, "time"=w478) -> ("error out"=w480:errorcluster)  [unwired: 1 out]
                        n154 = call <userlib>:"SetNumberKinetics.vi"("error in (no error)"=w480, "number"=w500) -> ("error out"=w504:errorcluster)  [unwired: 1 out]
                        n155 = call <userlib>:"SetSpool.vi"("active"=TRUE, "method"=Spool_method_typedef."16-buit TIFF", "name"=w497, "framebuffersize (10)"=10, "error in (no error)"=w504) -> ("error out"=w503:errorcluster)  [unwired: 9 in, 1 out]
                        n156 = call "shutter.vi"("error in (no error)"=w503, "Boolean"=TRUE, "lines"=w495) -> ("error out"=w505:errorcluster)  [unwired: 1 in]
                        n157 = call <userlib>:"StartAcquisition.vi"("error in (no error)"=w505) -> ("error out"=w482:errorcluster)  [unwired: 1 in, 1 out]
                      }
                      frame "Acquiring" {
                        # "Put waiting here so that the loop is less demanding in CPU resource."
                        n158 = call <userlib>:"GetTotalNumberImagesAcquired.vi"() -> ("index"=→"Current Frame":i32)  [unwired: 3 in, 2 out]
                        n159 = Multiply(x=w514, y=sgl 1000.0) -> (x*y=w516:sgl)
                        n160 = Add(x=w516, y=sgl 21.0) -> (x+y=w513:sgl)
                        n161 = Wait (ms)(milliseconds to wait=w513) -> ()  [unwired: 1 out]
                        n162 = call <userlib>:"GetMostRecentImage16.vi"("error in (no error)"=w529, "size"=w527, "array"=w528) -> ("error out"=w531:errorcluster, "array"=w535:u16[], "DLL error code"=w534:u32)
                        n163 = call <userlib>:"GetStatus.vi"("error in (no error)"=w531) -> ("error out"=w520:errorcluster, "status"=w533:T16)  [unwired: 2 in, 1 out]
                        n164 = Equal?(x=w523, y=w534) -> (x = y?=w536:bool)
                        n165 = Equal?(x=w533, y=72) -> (x = y?=w522:bool)
                        n166 = case shown="True" w536 {
                          tunnel: w535 -> [_ w552]
                          tunnel: w524 -> [_ w551]
                          tunnel: w525 -> [_ w550]
                          tunnel: w526 -> [_ w547]
                          frame False {
                          }
                          frame True {
                            n167 = Reshape Array(w552, w550, w551) -> (w549:u16[][])
                            n168 = call "IMAQ ArrayToImage"("Image Pixels (U16)"=w549, "Image"=w547) -> ("Image Out"=w548:T4)  [unwired: 8 in, 1 out]
                            n169 = local write "Image 3"(w548) -> ()
                          }
                        }
                        n170 = case shown="False" w522 {
                          selector: w522 -> [w542 w543]
                          tunnel: w521 -> [w541 _]
                          tunnel: w520 -> [w540 w546]
                          tunnel: [w539 w546] -> w519
                          tunnel: [w538 w544] -> w518
                          tunnel: [enum16{"Start", "Acquiring", "Acquiring2"}."Start" enum16{"Start", "Acquiring", "Acquiring2"}."Acquiring"] -> w517
                          frame False {
                            n171 = call "shutter.vi"("error in (no error)"=w540, "Boolean"=w542, "lines"=w541) -> ("error out"=w539:errorcluster)  [unwired: 1 in]
                            n172 = Not(x=w542) -> (.not. x?=w538:bool)
                          }
                          frame True {
                            n173 = Not(x=w543) -> (.not. x?=w544:bool)
                          }
                        }
                      }
                      frame "Acquiring2" {
                      }
                    }
                  }
                }
              }
              frame "TIRF-Coupled-Confocal" {
                # "TIRF-confocal acquisition would be performed iteratively until certain number of trajectory has been collected."
                n174 = case shown="\"Acquiring2\"" w562 {
                  tunnel: w582 -> [_ w639 _]
                  tunnel: w561 -> [w600 w641 w674]
                  tunnel: w569 -> [w592 _ _]
                  tunnel: w581 -> [_ _ _]
                  tunnel: w580 -> [_ w638 _]
                  tunnel: w579 -> [_ w637 _]
                  tunnel: w578 -> [_ w635 _]
                  tunnel: w577 -> [_ w636 _]
                  tunnel: w576 -> [w608 _ w735]
                  tunnel: w575 -> [w607 _ w734]
                  tunnel: w564 -> [w583 w654 w667]
                  tunnel: [w583 w654 w669] -> w565
                  tunnel: w574 -> [w618 _ w740]
                  tunnel: w573 -> [_ _ w738]
                  tunnel: w572 -> [_ _ w737]
                  tunnel: w571 -> [_ _ w687]
                  tunnel: w570 -> [_ _ w698]
                  tunnel: w568 -> [w593 w644 _]
                  tunnel: w566 -> [w598 _ _]
                  tunnel: [w589 w632 w670] -> w558
                  tunnel: [enum16{"Start", "Acquiring", "Acquiring2"}."Acquiring" w631 enum16{"Start", "Acquiring", "Acquiring2"}."Start"] -> w563
                  tunnel: w560 -> [_ w640 _]
                  tunnel: tag "6052E/port0/line0" ("lines") -> [w586 w630 _]
                  tunnel: w557 -> [_ _ w673]
                  tunnel: [FALSE FALSE w672] -> w556
                  tunnel: w555 -> [w584 _ _]
                  frame "Start" {
                    # "The \"start\" and \"Acquiring\" are the same as \"kinetics\" mode of camera data acquisition"
                    n175 = Format Value(format string="%d", value (0)=w583) -> (output string=w610:string)  [unwired: 1 in]
                    n176 = Concatenate Strings(w607, "." ("string"), w610) -> (w612:string)
                    n177 = case shown="False" w584 {
                      tunnel: w598 -> [w625 _]
                      tunnel: [w621 w626] -> w599
                      tunnel: w600 -> [w624 w626]
                      frame False {
                        n178 = invoke class="MG17Motor" method="MoveJog"(reference=w625, error in=w624, "lChanID"=0, "lJogDir"=1) -> (error out=w621:errorcluster)  [unwired: 1 in, 4 out]
                      }
                      frame True {
                      }
                    }
                    n179 = Build Path(base path=w608, name or relative path=w612) -> (appended path=w606:path)
                    n180 = Path To String(path=w606) -> (string=w605:string)
                    n181 = invoke class="MG17Motor" method="MoveJog"(reference=w618, error in=w599, "lChanID"=0, "lJogDir"=2) -> (error out=w616:errorcluster)  [unwired: 1 in, 4 out]
                    n182 = flat-sequence {
                      tunnel: w616 -> [w627]
                      tunnel: [w627] -> w595
                      frame #0 {
                        n183 = Wait (ms)(milliseconds to wait=u32 1000) -> ()  [unwired: 1 out]
                      }
                    }
                    n184 = call <userlib>:"GetCameraHandle.vi"("error in (no error)"=w595, "cameraIndex"=0) -> ("error out"=w603:errorcluster, "cameraHandle"=w604:i32)  [unwired: 1 in, 1 out]
                    n185 = call <userlib>:"SetCurrentCamera.vi"("error in (no error)"=w603, "cameraHandle"=w604) -> ("error out"=w590:errorcluster)  [unwired: 1 out]
                    n186 = call <userlib>:"SetExposureTime.vi"("error in (no error)"=w590, "time"=w593) -> ("error out"=w594:errorcluster)  [unwired: 1 out]
                    n187 = call <userlib>:"SetAcquisitionMode.vi"("error in (no error)"=w594, "mode"=AcquisitionMode_mode_typedef."Kinetics") -> ("error out"=w601:errorcluster)  [unwired: 1 out]
                    n188 = call <userlib>:"SetNumberKinetics.vi"("error in (no error)"=w601, "number"=w592) -> ("error out"=w591:errorcluster)  [unwired: 1 out]
                    n189 = call <userlib>:"SetSpool.vi"("active"=TRUE, "method"=Spool_method_typedef."16-buit TIFF", "name"=w605, "framebuffersize (10)"=10, "error in (no error)"=w591) -> ("error out"=w615:errorcluster)  [unwired: 9 in, 1 out]
                    n190 = call "shutter.vi"("error in (no error)"=w615, "Boolean"=TRUE, "lines"=w586) -> ("error out"=w611:errorcluster)  [unwired: 1 in]
                    n191 = call <userlib>:"StartAcquisition.vi"("error in (no error)"=w611) -> ("error out"=w589:errorcluster)  [unwired: 1 in, 1 out]
                  }
                  frame "Acquiring" {
                    n192 = call <userlib>:"GetTotalNumberImagesAcquired.vi"() -> ("index"=w647:i32)  [unwired: 3 in, 2 out]
                    n193 = Multiply(x=w644, y=sgl 1000.0) -> (x*y=w646:sgl)
                    n194 = local write "Current Frame"(w647) -> ()
                    n195 = Add(x=w646, y=sgl 21.0) -> (x+y=w642:sgl)
                    n196 = Wait (ms)(milliseconds to wait=w642) -> ()  [unwired: 1 out]
                    n197 = call <userlib>:"GetMostRecentImage16.vi"("error in (no error)"=w641, "size"=w637, "array"=w638) -> ("error out"=w648:errorcluster, "array"=w650:u16[], "DLL error code"=w649:u32)
                    n198 = Equal?(x=w639, y=w649) -> (x = y?=w653:bool)
                    n199 = case shown="True" w653 {
                      tunnel: w650 -> [_ w666]
                      tunnel: w635 -> [_ w665]
                      tunnel: w636 -> [_ w664]
                      tunnel: w640 -> [_ w662]
                      frame False {
                      }
                      frame True {
                        n200 = Reshape Array(w666, w664, w665) -> (w663:u16[][])
                        n201 = call "IMAQ ArrayToImage"("Image Pixels (U16)"=w663, "Image"=w662) -> ("Image Out"=→"Image":T4)  [unwired: 8 in, 1 out]
                      }
                    }
                    n202 = call <userlib>:"GetStatus.vi"("error in (no error)"=w648) -> ("error out"=w633:errorcluster, "status"=w652:T16)  [unwired: 2 in, 1 out]
                    n203 = Equal?(x=w652, y=72) -> (x = y?=w634:bool)
                    n204 = case shown="False" w634 {
                      tunnel: w633 -> [w656 w660]
                      tunnel: [w655 w660] -> w632
                      tunnel: [enum16{"Start", "Acquiring", "Acquiring2"}."Acquiring2" enum16{"Start", "Acquiring", "Acquiring2"}."Acquiring"] -> w631
                      tunnel: w630 -> [w657 _]
                      frame False {
                        n205 = call "shutter.vi"("error in (no error)"=w656, "lines"=w657) -> ("error out"=w655:errorcluster)  [unwired: 2 in]
                      }
                      frame True {
                      }
                    }
                  }
                  frame "Acquiring2" {
                    w704 = u32 10 ("Nb pts X")
                    w714 = 0
                    w730 = T18 {"Objects"=0, "Threshold"=0, "Reject Border"=FALSE, "Fill Holes"=FALSE, "Min Object Size"=FALSE, "Min Size"=0, "Max Object Size"=FALSE, "Max Size"=0, "Show Search Area"=FALSE, "Show Center"=FALSE, "Show Bounding Box"=FALSE}  # Settings
                    # "This \"Terminate Trajectory\" is used to skip the current \ntrajectory manually."
                    # "A quicl rescan and gaussian fitting will be performed\naround the picked molecule. Can be enabled if it helps \nto improve the positioning accuracy. Here it is skipped."
                    # "signal-to-background ratio used as a threshold \nfor picking molecules."
                    # "The \"tif2image.vi\" is used to \nextract the last frame of the just-saved tiff data file containing certain number of frames."
                    # "\"Acquiring 2\" case take care of the confocal part."
                    # "stage move to the \ncalculated coordinate"
                    # "This subvi calculate the transformation of coordinate from TIRF to confocal."
                    # "Motorized mirror flip control the \nswitch to confocal mode"
                    # "Randomly pick one spot from all the detected\nonce and passed to confocal mode"
                    # "To choose which region of image would be \nused to identified spots."
                    # "The latest acquied image is loaded \nand analyzed by IMAQ function."
                    n206 = Format Value(format string="%d", value (0)=w667) -> (output string=w694:string)  [unwired: 1 in]
                    n207 = Concatenate Strings(w734, "." ("string"), w694, ".tif" ("string")) -> (w736:string)
                    n208 = Build Path(base path=w735, name or relative path=w736) -> (appended path=w682:path)
                    n209 = case shown="\"Entire Image\"" w687 {
                      tunnel: [T14 {"Left"=257, "Top"=0, "Right"=511, "Bottom"=511, "Rotation"=0.0} ("Rectangle") T14 {"Left"=0, "Top"=0, "Right"=250, "Bottom"=511, "Rotation"=0.0} ("Rectangle") T14 {"Left"=0, "Top"=0, "Right"=511, "Bottom"=511, "Rotation"=0.0} ("Rectangle")] -> w731
                      frame "Donor" {
                      }
                      frame "Acceptor" {
                      }
                      frame "Entire Image" {
                      }
                    }
                    n210 = call <userlib>:"libtiff3_tif2Images.vi"("error in (no error)"=w674, "Input path"=w682) -> ("error out"=w683:errorcluster, "ImageArray"=w678:T4[])  [unwired: 8 in]
                    n211 = Array Size(array=w678) -> (size(s)=w681:i32)
                    n212 = Decrement(x=w681) -> (x-1=w680:i32)
                    n213 = Index Array(array=w678, index=w680) -> (element=w679:T4)
                    n214 = case shown="\"Entire Image\"" w687 {
                      tunnel: [1.7 ("y") 1.6 ("y") 5.0 ("y")] -> w715
                      frame "Donor", Default {
                      }
                      frame "Acceptor" {
                      }
                      frame "Entire Image" {
                      }
                    }
                    n215 = Bundle(w714, w714) -> (→"Trajectory":cluster{i32, i32})  [unwired: 1 in]
                    n216 = call "IMAQ Light Meter (Rectangle)"("error in (no error)"=w683, "Rectangle"=w731, "Image"=w679) -> ("error out"=w732:errorcluster, "Gray Level Intensities"=w728:T19, "Image Out"=w733:T4)  [unwired: 4 in, 2 out]
                    n217 = Unbundle By Name(w728) -> ("Mean Intensity"=w716:sgl)
                    n218 = Multiply(x=w715, y=w716) -> (x*y=w727:dbl)
                    n219 = Bundle By Name(cluster=w730, "Objects"=u16 0, "Threshold"=w727, "Min Object Size"=TRUE, "Min Size"=4, "Max Object Size"=TRUE, "Max Size"=50, "Show Search Area"=TRUE, "Show Center"=FALSE, "Show Bounding Box"=TRUE) -> (w729:T18)
                    n220 = call "IMAQ Count Objects 2"("Settings"=w729, "error in (no error)"=w732, "Search Rect (entire image)"=w731, "Image"=w733) -> ("error out"=w718:errorcluster, "Image Out"=w684:T4, "Objects"=w720:T20)  [unwired: 3 in, 2 out]
                    n221 = invoke class="MG17Motor" method="MoveJog"(reference=w740, error in=w718, "lChanID"=0, "lJogDir"=1) -> (error out=w711:errorcluster)  [unwired: 1 in, 4 out]
                    n222 = property on="Trajectory" class="WFChart (strict)"("History Data"=cluster{i32, i32}[] []) -> ()  [unwired: 2 in, 2 out]
                    n223 = local write "Image"(w684) -> ()
                    n224 = for {
                      shift-right: [w786] -> w717
                      shift-left: cluster{"X":sgl, "Y":sgl}[] [] -> [w785]
                      tunnel: w720 -> [w784] mode=indexing
                      n225 = Unbundle By Name(w784) -> ("Object Center"=w787:cluster{"X":sgl, "Y":sgl})  [unwired: 5 out]
                      n226 = Build Array (concatenate)(w785, w787) -> (w786:cluster{"X":sgl, "Y":sgl}[])
                    }
                    n227 = control-ref of="Trajectory"() -> (w692:refnum<vi>)
                    n228 = control-ref of="Terminate Trajectory"() -> (w697:refnum<vi>)
                    n229 = Format Value(format string="%d", value (0)=w667) -> (output string=w701:string)  [unwired: 1 in]
                    n230 = Increment(x=w667) -> (x+1=w669:u32)
                    "Current Traj#" <- w669
                    n231 = Build Path(base path=w735, name or relative path=w701) -> (appended path=w700:path)
                    n232 = Array Size(array=w717) -> (size(s)=w744:i32)
                    n233 = Random Number (0-1)() -> (number: 0 to 1=w743:dbl)
                    n234 = Greater Or Equal?(x=w669, y=w673) -> (x >= y?=w672:bool)
                    n235 = Multiply(x=w744, y=w743) -> (x*y=w742:dbl)
                    n236 = Round To Nearest(number=w742) -> (nearest integer value=w741:dbl)
                    "Spot Index" <- w741
                    n237 = Index Array(array=w717, index=w741) -> (element=w686:cluster{"X":sgl, "Y":sgl})
                    "Spot Center" <- w686
                    n238 = Unbundle By Name(w686) -> ("X"=w689:sgl, "Y"=w739:sgl)
                    n239 = case shown="\"Entire Image\"" w687 {
                      tunnel: w689 -> [w747 w752 w753]
                      tunnel: [w748 w750 w754] -> w688
                      frame "Donor", Default {
                        n240 = Subtract(x=w747, y=sgl 128.0) -> (x-y=w748:sgl)
                      }
                      frame "Acceptor" {
                        n241 = Add(x=w752, y=sgl 128.0) -> (x+y=w750:sgl)
                      }
                      frame "Entire Image" {
                        n242 = Subtract(x=w753, y=sgl 0.0) -> (x-y=w754:sgl)
                      }
                    }
                    n243 = call "tform_t2c.vi"("X_TIRF"=w688, "Y_TIRF"=w739, "X_Stage"=w738, "Y_Stage"=w737, "Nb pts X&Y"=w704) -> ("Scanning parameters"=w707:T21, "Y_cfc"=w705:dbl, "X_cfc"=w706:dbl)  [unwired: 11 in, 1 out]
                    n244 = case shown="True" FALSE ("Rescan?") {
                      tunnel: w711 -> [w764 w775]
                      tunnel: [w764 w772] -> w710
                      tunnel: [w763 w771] -> w709
                      tunnel: [w762 w770] -> w708
                      tunnel: w707 -> [_ w769]
                      tunnel: w706 -> [w758 w766]
                      tunnel: w705 -> [w757 w767]
                      tunnel: w704 -> [_ w768]
                      frame False {
                        w756 = 0
                        w761 = 0.1
                        n245 = Add(x=w756, y=w757) -> (x+y=w760:dbl)
                        n246 = Add(x=w756, y=w758) -> (x+y=w759:dbl)
                        n247 = Multiply(x=w760, y=w761) -> (x*y=w763:dbl)
                        n248 = Multiply(x=w759, y=w761) -> (x*y=w762:dbl)
                      }
                      frame True {
                        n249 = call "APDStageScan.vi"("error in (no error)"=w775, "Scanning parameters"=w769) -> ("error out"=w774:errorcluster, "output array"=w773:u32[][])  [unwired: 2 in]
                        n250 = call "2DGaussianFit.vi"("error in (no error)"=w774, "Nb Pts X&Y"=w768, "Input Image Array"=w773) -> ("error out"=w772:errorcluster, "Best Fit"=w765:dbl[])  [unwired: 1 out]
                        n251 = call "cfc_center.vi"("Fitted Pos"=w765, "Nb pts X&Y"=w768, "X_cfc"=w766, "Y_cfc"=w767) -> ("X volt"=w771:dbl, "Y volt"=w770:dbl)  [unwired: 2 in, 1 out]
                      }
                    }
                    n252 = Merge Signals(w708, w709) -> (w703:dynamicdata)
                    n253 = call "AO X&Y"("data"=w703, "error in"=w710) -> ("error out"=w699:errorcluster)  [unwired: 16 in, 1 out]
                    n254 = case shown="True" TRUE {
                      tunnel: w700 -> [_ w783]
                      tunnel: w699 -> [w776 w782]
                      tunnel: w692 -> [_ w781]
                      tunnel: w698 -> [_ w780]
                      tunnel: w697 -> [_ w779]
                      tunnel: [w776 w778] -> w671
                      frame False {
                      }
                      frame True {
                        # "confocal data acquisition\nfrom APDs"
                        n255 = call "cfcAPDtraj.vi"("file path (use dialog)"=w783, "Save Trajectory?"=TRUE, "Trajectory length (s)"=w780, "FRET Refnum"=w781, "Stop Refnum"=w779, "error in (no error)"=w782) -> ("error out"=w778:errorcluster)  [unwired: 1 in, 1 out]
                      }
                    }
                    n256 = flat-sequence {
                      tunnel: w671 -> [w745]
                      tunnel: [w745] -> w670
                      frame #0 {
                        n257 = Wait (ms)(milliseconds to wait=u32 1000) -> ()  [unwired: 1 out]
                      }
                    }
                  }
                }
                n258 = local write "Illumination Mode"(enum16{"TIRF", "Dark-Field"}."TIRF" ("Illumination Mode")) -> ()
                n259 = property on="Save Button" class="Bool"("DisabledEnum"=T12."Disabled and Grayed Out" ("Disabled")) -> ()  [unwired: 2 in, 2 out]
              }
              frame "Imaging Spectrograph" {
                # "Settings for camera is similar as in \"wide-field imaging\" case. \nSettings for monochromator/spectrograph itself is not included here \nsince in many case those settings does not need to be changed."
                n260 = case shown="\"TIRF\"" w813 {
                  tunnel: [tag "6052E/port0/line0" ("lines") tag "6602/port0/line6" ("lines")] -> w812
                  frame "TIRF" {
                  }
                  frame "Dark-Field" {
                  }
                }
                n261 = case shown="\"Live Monitoring\"" "Camera DAQ Mode 2" {
                  tunnel: w817 -> [w819 _]
                  tunnel: w816 -> [w840 _]
                  tunnel: w815 -> [w839 _]
                  tunnel: w814 -> [w836 w884]
                  tunnel: w794 -> [w835 w885]
                  tunnel: w812 -> [w834 w867]
                  tunnel: w811 -> [w827 w886]
                  tunnel: w810 -> [w826 w883]
                  tunnel: [w824 w876] -> w809
                  tunnel: w807 -> [w823 w870]
                  tunnel: "Exposure Time(s) 2" -> [w821 w882]
                  tunnel: "Number of Frames to Acquire 2" -> [_ w881]
                  tunnel: w804 -> [_ w879]
                  tunnel: w803 -> [_ w878]
                  tunnel: w802 -> [_ w875]
                  tunnel: [_ w874] -> w801
                  tunnel: w800 -> [_ w873]
                  tunnel: w799 -> [_ w872]
                  tunnel: w798 -> [_ w871]
                  tunnel: w797 -> [_ w869]
                  tunnel: w796 -> [_ w868]
                  tunnel: [FALSE w866] -> w795
                  frame "Live Monitoring" {
                    n262 = invoke class="MG17Motor" method="MoveJog"(reference=w826, error in=w827, "lChanID"=0, "lJogDir"=2) -> (error out=w825:errorcluster)  [unwired: 1 in, 4 out]
                    n263 = property on="Save Button" class="Bool"("DisabledEnum"=T12."Enabled" ("Disabled")) -> ()  [unwired: 2 in, 2 out]
                    n264 = case shown="False" w835 {
                      tunnel: w836 -> [w856 _]
                      tunnel: [w857 w860] -> w831
                      tunnel: w825 -> [w855 w860]
                      frame False {
                        n265 = invoke class="MG17Motor" method="MoveJog"(reference=w856, error in=w855, "lChanID"=0, "lJogDir"=2) -> (error out=w857:errorcluster)  [unwired: 1 in, 4 out]
                      }
                      frame True {
                      }
                    }
                    n266 = call <userlib>:"GetCameraHandle.vi"("error in (no error)"=w831, "cameraIndex"=1) -> ("error out"=w832:errorcluster, "cameraHandle"=w833:i32)  [unwired: 1 in, 1 out]
                    n267 = call <userlib>:"SetCurrentCamera.vi"("error in (no error)"=w832, "cameraHandle"=w833) -> ("error out"=w830:errorcluster)  [unwired: 1 out]
                    n268 = call <userlib>:"SetExposureTime.vi"("error in (no error)"=w830, "time"=w821) -> ("error out"=w841:errorcluster)  [unwired: 1 out]
                    n269 = call <userlib>:"SetAcquisitionMode.vi"("error in (no error)"=w841, "mode"=AcquisitionMode_mode_typedef."Single Scan") -> ("error out"=w850:errorcluster)  [unwired: 1 out]
                    n270 = call <userlib>:"SetSpool.vi"("active"=FALSE, "method"=Spool_method_typedef."16-buit TIFF", "name"="", "error in (no error)"=w850) -> ("error out"=w849:errorcluster)  [unwired: 10 in, 1 out]
                    n271 = call "shutter.vi"("error in (no error)"=w849, "Boolean"=TRUE, "lines"=w834) -> ("error out"=w852:errorcluster)  [unwired: 1 in]
                    n272 = call <userlib>:"StartAcquisition.vi"("error in (no error)"=w852) -> ("error out"=w854:errorcluster)  [unwired: 1 in, 1 out]
                    n273 = while {
                      tunnel: w854 -> [w863]
                      tunnel: [w865] -> w845
                      stop <- w861 continue-if-true
                      n274 = call <userlib>:"GetStatus.vi"("error in (no error)"=w863) -> ("error out"=w865:errorcluster, "status"=w862:T16)  [unwired: 2 in, 1 out]
                      n275 = Equal?(x=w862, y=72) -> (x = y?=w861:bool)
                    }
                    n276 = call <userlib>:"GetAcquiredData16.vi"("error in (no error)"=w845, "size"=w819) -> ("error out"=w824:errorcluster, "array"=w844:u16[])  [unwired: 1 in, 1 out]
                    n277 = Multiply(x=w844, y=1) -> (x*y=w842:i32[])
                    n278 = Reshape Array(w842, w840, w839) -> (w838:i32[][])
                    n279 = call "IMAQ ArrayToImage"("Image Pixels (U16)"=w838, "Image"=w823) -> ("Image Out"=→"Image 2":T4)  [unwired: 8 in, 1 out]
                  }
                  frame "Kinetics Series Scan" {
                    n280 = Build Path(base path=w879, name or relative path=w878) -> (appended path=w880:path)
                    n281 = Path To String(path=w880) -> (string=w877:string)
                    n282 = case shown="\"Start\"" w875 {
                      tunnel: w886 -> [w900 w939 w964]
                      tunnel: w885 -> [w899 _ _]
                      tunnel: w884 -> [w898 _ _]
                      tunnel: w883 -> [w897 _ _]
                      tunnel: w882 -> [w896 w932 _]
                      tunnel: w881 -> [w895 _ _]
                      tunnel: w877 -> [w894 _ _]
                      tunnel: [w893 w935 w964] -> w876
                      tunnel: [enum16{"Start", "Acquiring", "Acquiring2"}."Acquiring" w925 _] -> w874
                      tunnel: w873 -> [_ w938 _]
                      tunnel: w872 -> [_ w934 _]
                      tunnel: w871 -> [_ w933 _]
                      tunnel: w870 -> [_ w930 _]
                      tunnel: w869 -> [_ w928 _]
                      tunnel: w868 -> [_ w927 _]
                      tunnel: w867 -> [w888 w924 _]
                      tunnel: [FALSE w923 _] -> w866
                      frame "Start" {
                        # "open shutter"
                        n283 = invoke class="MG17Motor" method="MoveJog"(reference=w897, error in=w900, "lChanID"=0, "lJogDir"=2) -> (error out=w901:errorcluster)  [unwired: 1 in, 4 out]
                        n284 = property on="Save Button" class="Bool"("DisabledEnum"=T12."Disabled and Grayed Out" ("Disabled")) -> ()  [unwired: 2 in, 2 out]
                        n285 = case shown="False" w899 {
                          tunnel: w898 -> [w918 _]
                          tunnel: [w919 w922] -> w904
                          tunnel: w901 -> [w917 w922]
                          frame False {
                            n286 = invoke class="MG17Motor" method="MoveJog"(reference=w918, error in=w917, "lChanID"=0, "lJogDir"=2) -> (error out=w919:errorcluster)  [unwired: 1 in, 4 out]
                          }
                          frame True {
                          }
                        }
                        n287 = call <userlib>:"GetCameraHandle.vi"("error in (no error)"=w904, "cameraIndex"=1) -> ("error out"=w905:errorcluster, "cameraHandle"=w906:i32)  [unwired: 1 in, 1 out]
                        n288 = call <userlib>:"SetCurrentCamera.vi"("error in (no error)"=w905, "cameraHandle"=w906) -> ("error out"=w890:errorcluster)  [unwired: 1 out]
                        n289 = call <userlib>:"SetAcquisitionMode.vi"("error in (no error)"=w890, "mode"=AcquisitionMode_mode_typedef."Kinetics") -> ("error out"=w907:errorcluster)  [unwired: 1 out]
                        n290 = call <userlib>:"SetExposureTime.vi"("error in (no error)"=w907, "time"=w896) -> ("error out"=w908:errorcluster)  [unwired: 1 out]
                        n291 = call <userlib>:"SetNumberKinetics.vi"("error in (no error)"=w908, "number"=w895) -> ("error out"=w915:errorcluster)  [unwired: 1 out]
                        n292 = call <userlib>:"SetSpool.vi"("active"=TRUE, "method"=Spool_method_typedef."16-buit TIFF", "name"=w894, "framebuffersize (10)"=10, "error in (no error)"=w915) -> ("error out"=w914:errorcluster)  [unwired: 9 in, 1 out]
                        n293 = call "shutter.vi"("error in (no error)"=w914, "Boolean"=TRUE, "lines"=w888) -> ("error out"=w916:errorcluster)  [unwired: 1 in]
                        n294 = call <userlib>:"StartAcquisition.vi"("error in (no error)"=w916) -> ("error out"=w893:errorcluster)  [unwired: 1 in, 1 out]
                      }
                      frame "Acquiring" {
                        n295 = Multiply(x=w932, y=sgl 1000.0) -> (x*y=w943:sgl)
                        n296 = Add(x=w943, y=sgl 21.0) -> (x+y=w941:sgl)
                        n297 = call <userlib>:"GetTotalNumberImagesAcquired.vi"() -> ("index"=→"Current Frame 2":i32)  [unwired: 3 in, 2 out]
                        n298 = Wait (ms)(milliseconds to wait=w941) -> ()  [unwired: 1 out]
                        n299 = call <userlib>:"GetMostRecentImage16.vi"("error in (no error)"=w939, "size"=w933, "array"=w934) -> ("error out"=w944:errorcluster, "array"=w929:u16[], "DLL error code"=w947:u32)
                        n300 = call <userlib>:"GetStatus.vi"("error in (no error)"=w944) -> ("error out"=w937:errorcluster, "status"=w946:T16)  [unwired: 2 in, 1 out]
                        n301 = Equal?(x=w938, y=w947) -> (x = y?=w926:bool)
                        n302 = case shown="True" w926 {
                          tunnel: w930 -> [_ w952]
                          tunnel: w929 -> [_ w951]
                          tunnel: w928 -> [_ w949]
                          tunnel: w927 -> [_ w948]
                          frame False {
                          }
                          frame True {
                            n303 = Reshape Array(w951, w949, w948) -> (w953:u16[][])
                            n304 = call "IMAQ ArrayToImage"("Image Pixels (U16)"=w953, "Image"=w952) -> ("Image Out"=w950:T4)  [unwired: 8 in, 1 out]
                            n305 = local write "Image 2"(w950) -> ()
                          }
                        }
                        n306 = Equal?(x=w946, y=72) -> (x = y?=w936:bool)
                        n307 = case shown="False" w936 {
                          selector: w936 -> [w955 w960]
                          tunnel: w937 -> [w959 w962]
                          tunnel: [w958 w962] -> w935
                          tunnel: [enum16{"Start", "Acquiring", "Acquiring2"}."Start" enum16{"Start", "Acquiring", "Acquiring2"}."Acquiring"] -> w925
                          tunnel: w924 -> [w956 _]
                          tunnel: [w954 w961] -> w923
                          frame False {
                            n308 = call "shutter.vi"("error in (no error)"=w959, "Boolean"=w955, "lines"=w956) -> ("error out"=w958:errorcluster)  [unwired: 1 in]
                            n309 = Not(x=w955) -> (.not. x?=w954:bool)
                          }
                          frame True {
                            n310 = Not(x=w960) -> (.not. x?=w961:bool)
                          }
                        }
                      }
                      frame "Acquiring2" {
                      }
                    }
                  }
                }
              }
            }
            n311 = Not(x="Start") -> (.not. x?=w331:bool)
            n312 = local write "Ready"(w331) -> ()
            n313 = case shown="False" "Start" {
              tunnel: [-1 0] -> w358
              frame False {
                n314 = call "shutter.vi"("Boolean"=FALSE, "lines"=tag "6052E/port0/line0") -> ()  [unwired: 2 in, 1 out]
                n315 = call "shutter.vi"("Boolean"=FALSE, "lines"=tag "6602/port0/line6") -> ()  [unwired: 2 in, 1 out]
              }
              frame True {
              }
            }
            n316 = case shown="True" w354 {
              selector: w354 -> [_ w373]
              tunnel: w358 -> [w371 _]
              tunnel: [w371 -1] -> w357
              tunnel: w356 -> [w372 w377]
              tunnel: [w372 w377] -> w355
              frame False {
                n317 = property on="Ready" class="Bool (strict)"("Blinking"=TRUE) -> ()  [unwired: 2 in, 2 out]
                n318 = property on="Ready" class="Bool (strict)"("Caption.Text"="Acquring") -> ()  [unwired: 2 in, 2 out]
              }
              frame True {
                n319 = Not(x=w373) -> (.not. x?=w374:bool)
                n320 = local write "Ready"(w373) -> ()
                n321 = property on="Ready" class="Bool (strict)"("Blinking"=w374) -> ()  [unwired: 2 in, 2 out]
                n322 = property on="Ready" class="Bool (strict)"("Caption.Text"="Ready") -> ()  [unwired: 2 in, 2 out]
                n323 = local write "Start"(w374) -> ()
              }
            }
          }
          event "Save Button": Value Change {
            # "Save one image frame with specified file name to the selected path."
            n324 = event-data() -> ()  [unwired: 1 in, 6 out]
            n325 = local read "Data Saving Path"() -> (w970:path)
            n326 = call "File Dialog"("start path"=w970) -> ("selected path"=w969:path, "error out"=w968:errorcluster)  [unwired: 11 in, 2 out]
            n327 = Path To String(path=w969) -> (string=w971:string)
            n328 = call <userlib>:"SaveAsTiff.vi"("path"=w971, "palette"="", "position"=1, "type"=Tiff_type_typedef."16-bit", "error in (no error)"=w968) -> ()  [unwired: 9 in, 2 out]
          }
          event "Stop": Value Change {
            w979 = FALSE
            n329 = event-data() -> ()  [unwired: 1 in, 6 out]
            n330 = local read "Illumination Mode"() -> (w978:enum16{"TIRF", "Dark-Field"})
            n331 = case shown="\"TIRF\"" w978 {
              tunnel: [tag "6052E/port0/line0" ("lines") tag "6602/port0/line6" ("lines")] -> w977
              frame "TIRF" {
              }
              frame "Dark-Field" {
              }
            }
            n332 = property on="Ready" class="Bool (strict)"("Blinking"=FALSE) -> ()  [unwired: 2 in, 2 out]
            n333 = property on="Ready" class="Bool (strict)"("Caption.Text"="Ready") -> ()  [unwired: 2 in, 2 out]
            n334 = call "shutter.vi"("Boolean"=FALSE, "lines"=w977) -> ()  [unwired: 2 in, 1 out]
            n335 = call <userlib>:"AbortAcquisition.vi"() -> ()  [unwired: 2 in, 2 out]
            n336 = Not(x=w979) -> (.not. x?=w982:bool)
            n337 = local write "Start"(w979) -> ()
            n338 = local write "Ready"(w982) -> ()
          }
          event "System Shut Down": Value Change {
            w985 = T12."Enabled" ("Disabled")
            n339 = event-data() -> ()  [unwired: 1 in, 6 out]
            n340 = Not(x=w986) -> (.not. x?=w991:bool)
            n341 = Not(x=w988) -> (.not. x?=w992:bool)
            n342 = And(x=w992, y=w991) -> (x .and. y?=w990:bool)
            n343 = case shown="True" w990 {
              tunnel: w995 -> [w1007 w1022]
              tunnel: w994 -> [w1006 w1023]
              tunnel: [w1005 w1020] -> w993
              tunnel: w989 -> [w1004 w1021]
              tunnel: w986 -> [w996 _]
              frame False {
                n344 = case shown="True" w996 {
                  tunnel: w1004 -> [_ w1010]
                  frame False {
                  }
                  frame True {
                    n345 = invoke class="MG17Motor" method="StopCtrl"(reference=w1010) -> ()  [unwired: 2 in, 3 out]
                  }
                }
                n346 = invoke class="MG17Motor" method="StopCtrl"(reference=w1007) -> (error out=w997:errorcluster)  [unwired: 2 in, 2 out]
                n347 = call <userlib>:"CoolerOFF.vi"("error in (no error)"=w997) -> ("error out"=w998:errorcluster)  [unwired: 1 in, 1 out]
                n348 = call <userlib>:"IsInternalMechanicalShutter.vi"("error in (no error)"=w998) -> ("error out"=w1003:errorcluster, "InternalShutter"=w1001:i32)  [unwired: 2 in, 1 out]
                n349 = Equal?(x=w1001, y=1) -> (x = y?=w1002:bool)
                n350 = case shown="True" w1002 {
                  tunnel: w1003 -> [w1011 w1015]
                  tunnel: [w1011 w1014] -> w999
                  frame False {
                  }
                  frame True {
                    n351 = call <userlib>:"SetShutter.vi"("type"=Shutter_type_typedef."TTL High", "mode"=Shutter_mode_typedef."Close", "error in (no error)"=w1015) -> ("error out"=w1014:errorcluster)  [unwired: 11 in, 1 out]
                  }
                }
                n352 = call <userlib>:"ShutDown.vi"("error in (no error)"=w999) -> ("DLL error code"=w1008:u32)  [unwired: 1 in, 1 out]
                n353 = Equal?(x=w1006, y=w1008) -> (x = y?=w1009:bool)
                n354 = case shown="True" w1009 {
                  tunnel: [TRUE w1019] -> w1005
                  frame False {
                    n355 = One Button Dialog(message="Shut Down Error") -> ()  [unwired: 1 in, 1 out]
                  }
                  frame True {
                    w1018 = FALSE
                    n356 = local write "Camera On"(w1018) -> ()
                    n357 = Not(x=w1018) -> (.not. x?=w1019:bool)
                    n358 = local write "Camera On 2"(w1018) -> ()
                    n359 = local write "Ready"(w1018) -> ()
                  }
                }
              }
              frame True {
                n360 = stacked-sequence {
                  tunnel: w1023 -> [w1028 w1056]
                  tunnel: w1022 -> [_ w1054]
                  tunnel: w1021 -> [w1026 _]
                  tunnel: [_ w1046] -> w1020
                  frame #0 {
                    n361 = invoke class="MG17Motor" method="StopCtrl"(reference=w1026) -> (error out=w1024:errorcluster)  [unwired: 2 in, 2 out]
                    n362 = call <userlib>:"GetCameraHandle.vi"("error in (no error)"=w1024, "cameraIndex"=1) -> ("error out"=w1038:errorcluster, "cameraHandle"=w1037:i32)  [unwired: 1 in, 1 out]
                    n363 = call <userlib>:"SetCurrentCamera.vi"("error in (no error)"=w1038, "cameraHandle"=w1037) -> ("error out"=w1035:errorcluster)  [unwired: 1 out]
                    n364 = call <userlib>:"CoolerOFF.vi"("error in (no error)"=w1035) -> ("error out"=w1025:errorcluster)  [unwired: 1 in, 1 out]
                    n365 = call <userlib>:"IsInternalMechanicalShutter.vi"("error in (no error)"=w1025) -> ("error out"=w1033:errorcluster, "InternalShutter"=w1031:i32)  [unwired: 2 in, 1 out]
                    n366 = Equal?(x=w1031, y=1) -> (x = y?=w1032:bool)
                    n367 = case shown="True" w1032 {
                      tunnel: w1033 -> [w1041 w1045]
                      tunnel: [w1041 w1044] -> w1029
                      frame False {
                      }
                      frame True {
                        n368 = call <userlib>:"SetShutter.vi"("type"=Shutter_type_typedef."TTL High", "mode"=Shutter_mode_typedef."Close", "error in (no error)"=w1045) -> ("error out"=w1044:errorcluster)  [unwired: 11 in, 1 out]
                      }
                    }
                    n369 = call <userlib>:"ShutDown.vi"("error in (no error)"=w1029) -> ("DLL error code"=w1034:u32)  [unwired: 1 in, 1 out]
                    n370 = Equal?(x=w1028, y=w1034) -> (x = y?=w1027:bool)
                    n371 = case shown="True" w1027 {
                      frame False {
                        n372 = One Button Dialog(message="Shut Down Error") -> ()  [unwired: 1 in, 1 out]
                      }
                      frame True {
                        w1040 = FALSE
                        n373 = local write "Camera On 2"(w1040) -> ()
                        n374 = local write "Ready"(w1040) -> ()
                      }
                    }
                  }
                  frame #1 {
                    n375 = invoke class="MG17Motor" method="StopCtrl"(reference=w1054) -> (error out=w1055:errorcluster)  [unwired: 2 in, 2 out]
                    n376 = call <userlib>:"GetCameraHandle.vi"("error in (no error)"=w1055, "cameraIndex"=0) -> ("error out"=w1061:errorcluster, "cameraHandle"=w1060:i32)  [unwired: 1 in, 1 out]
                    n377 = call <userlib>:"SetCurrentCamera.vi"("error in (no error)"=w1061, "cameraHandle"=w1060) -> ("error out"=w1057:errorcluster)  [unwired: 1 out]
                    n378 = call <userlib>:"CoolerOFF.vi"("error in (no error)"=w1057) -> ("error out"=w1047:errorcluster)  [unwired: 1 in, 1 out]
                    n379 = call <userlib>:"IsInternalMechanicalShutter.vi"("error in (no error)"=w1047) -> ("error out"=w1052:errorcluster, "InternalShutter"=w1050:i32)  [unwired: 2 in, 1 out]
                    n380 = Equal?(x=w1050, y=1) -> (x = y?=w1051:bool)
                    n381 = case shown="True" w1051 {
                      tunnel: w1052 -> [w1062 w1066]
                      tunnel: [w1062 w1065] -> w1048
                      frame False {
                      }
                      frame True {
                        n382 = call <userlib>:"SetShutter.vi"("type"=Shutter_type_typedef."TTL High", "mode"=Shutter_mode_typedef."Close", "error in (no error)"=w1066) -> ("error out"=w1065:errorcluster)  [unwired: 11 in, 1 out]
                      }
                    }
                    n383 = call <userlib>:"ShutDown.vi"("error in (no error)"=w1048) -> ("DLL error code"=w1058:u32)  [unwired: 1 in, 1 out]
                    n384 = Equal?(x=w1056, y=w1058) -> (x = y?=w1053:bool)
                    n385 = case shown="True" w1053 {
                      tunnel: [TRUE w1069] -> w1046
                      frame False {
                        n386 = One Button Dialog(message="Shut Down Error") -> ()  [unwired: 1 in, 1 out]
                      }
                      frame True {
                        w1070 = FALSE
                        n387 = Not(x=w1070) -> (.not. x?=w1069:bool)
                        n388 = local write "Camera On"(w1070) -> ()
                        n389 = local write "Ready"(w1070) -> ()
                      }
                    }
                  }
                }
              }
            }
            n390 = property on="Detection Mode" class="Enum (strict)"("Disabled Items []"=i32[] []) -> ()  [unwired: 2 in, 2 out]
            n391 = property on="Number of Traj to Acquire" class="DigNum (strict)"("DisabledEnum"=w985) -> ()  [unwired: 2 in, 2 out]
            n392 = property on="Spot Choosing Region" class="Enum (strict)"("DisabledEnum"=w985) -> ()  [unwired: 2 in, 2 out]
            n393 = property on="Trajectory Length (s)" class="DigNum (strict)"("DisabledEnum"=w985) -> ()  [unwired: 2 in, 2 out]
            n394 = property on="Cooling" class="Bool (strict)"("DisabledEnum"=w985) -> ()  [unwired: 2 in, 2 out]
            n395 = property on="Camera On" class="Bool (strict)"("DisabledEnum"=w985) -> ()  [unwired: 2 in, 2 out]
            n396 = property on="Current T(°C)" class="DigNum (strict)"("DisabledEnum"=w985) -> ()  [unwired: 2 in, 2 out]
            n397 = property on="Current T(°C) 2" class="DigNum (strict)"("DisabledEnum"=w985) -> ()  [unwired: 2 in, 2 out]
            n398 = property on="Camera On 2" class="Bool (strict)"("DisabledEnum"=w985) -> ()  [unwired: 2 in, 2 out]
            n399 = property on="Cooling 2" class="Bool (strict)"("DisabledEnum"=w985) -> ()  [unwired: 2 in, 2 out]
            n400 = property on="Current Frame 2" class="DigNum (strict)"("DisabledEnum"=w985) -> ()  [unwired: 2 in, 2 out]
            n401 = property on="Save Button" class="Bool"("DisabledEnum"=w985) -> ()  [unwired: 2 in, 2 out]
          }
          event "Quit Program": Value Change {
            w1071 = T12."Enabled" ("Disabled")
            w1072 = FALSE
            # "Re-enable all the controls"
            n402 = event-data() -> ()  [unwired: 1 in, 6 out]
            n403 = property on="Detection Mode" class="Enum (strict)"("Disabled Items []"=i32[] []) -> ()  [unwired: 2 in, 2 out]
            n404 = property on="Number of Traj to Acquire" class="DigNum (strict)"("DisabledEnum"=w1071) -> ()  [unwired: 2 in, 2 out]
            n405 = property on="Spot Choosing Region" class="Enum (strict)"("DisabledEnum"=w1071) -> ()  [unwired: 2 in, 2 out]
            n406 = property on="Trajectory Length (s)" class="DigNum (strict)"("DisabledEnum"=w1071) -> ()  [unwired: 2 in, 2 out]
            n407 = local write "Camera On"(w1072) -> ()
            n408 = Not(x=w1072) -> (.not. x?=w1074:bool)
            n409 = property on="Cooling" class="Bool (strict)"("DisabledEnum"=w1071) -> ()  [unwired: 2 in, 2 out]
            n410 = property on="Camera On" class="Bool (strict)"("DisabledEnum"=w1071) -> ()  [unwired: 2 in, 2 out]
            n411 = property on="Current T(°C)" class="DigNum (strict)"("DisabledEnum"=w1071) -> ()  [unwired: 2 in, 2 out]
            n412 = local write "Camera On 2"(w1072) -> ()
            n413 = local write "Ready"(w1072) -> ()
            n414 = property on="Current T(°C) 2" class="DigNum (strict)"("DisabledEnum"=w1071) -> ()  [unwired: 2 in, 2 out]
            n415 = property on="Camera On 2" class="Bool (strict)"("DisabledEnum"=w1071) -> ()  [unwired: 2 in, 2 out]
            n416 = property on="Cooling 2" class="Bool (strict)"("DisabledEnum"=w1071) -> ()  [unwired: 2 in, 2 out]
            n417 = property on="Current Frame 2" class="DigNum (strict)"("DisabledEnum"=w1071) -> ()  [unwired: 2 in, 2 out]
            n418 = property on="Save Button" class="Bool"("DisabledEnum"=w1071) -> ()  [unwired: 2 in, 2 out]
          }
        }
      }
      n419 = while {
        shift-right: [w217] -> _
        shift-left: 1000 -> [w218]
        tunnel: w177 -> [w216]
        tunnel: w176 -> [w215]
        shift-right: [w212] -> _
        shift-left: w175 -> [w214]
        shift-right: [w210] -> _
        shift-left: w175 -> [w209]
        stop <- w219 stop-if-true
        n420 = event shown="[0] Timeout" {
          selector: _ -> [_ _ _ _ _]
          dyn-events: _ -> [_ _ _ _ _]
          timeout: w218 -> [_ _ _ _ _]
          tunnel: [_ _ _ w292 w294] -> w219
          tunnel: [_ -1 1000 _ _] -> w217
          tunnel: w216 -> [w228 _ _ _ _]
          tunnel: w215 -> [w227 _ _ _ _]
          tunnel: w214 -> [w222 _ _ _ _]
          tunnel: "Camera T(°C)" -> [w226 _ _ _ _]
          tunnel: [w224 _ _ _ _] -> w212
          tunnel: "Camera T(°C)  2" -> [w225 _ _ _ _]
          tunnel: [w223 _ _ _ _] -> w210
          tunnel: w209 -> [w221 _ _ _ _]
          tunnel: "Cooling On" -> [w220 _ _ _ _]
          event Timeout {
            n421 = event-data() -> ()  [unwired: 1 in, 3 out]
            n422 = case shown="True" w220 {
              tunnel: w228 -> [_ w238]
              tunnel: w227 -> [_ w237]
              tunnel: w226 -> [_ w236]
              tunnel: w225 -> [_ w235]
              tunnel: [w230 w234] -> w224
              tunnel: [w229 w233] -> w223
              tunnel: w222 -> [w230 w232]
              tunnel: w221 -> [w229 w231]
              frame False {
              }
              frame True {
                n423 = stacked-sequence {
                  tunnel: w238 -> [w242 _]
                  tunnel: w237 -> [_ w267]
                  tunnel: w236 -> [w241 _]
                  tunnel: w235 -> [_ w266]
                  tunnel: [w240 _] -> w234
                  tunnel: [_ w265] -> w233
                  tunnel: w232 -> [w239 _]
                  tunnel: w231 -> [_ w264]
                  frame #0 {
                    n424 = case shown="False" w242 {
                      tunnel: w241 -> [w245 _]
                      tunnel: w239 -> [w244 _]
                      tunnel: [w243 _] -> w240
                      frame False {
                        n425 = case shown="\"Cooling\"" w244 {
                          tunnel: w245 -> [w247 w255]
                          tunnel: [enum16{"Start Cooling", "Cooling"}."Cooling" enum16{"Start Cooling", "Cooling"}."Cooling"] -> w243
                          frame "Start Cooling" {
                            n426 = call <userlib>:"GetCameraHandle.vi"("cameraIndex"=0) -> ("error out"=w250:errorcluster, "cameraHandle"=w251:i32)  [unwired: 2 in, 1 out]
                            n427 = call <userlib>:"SetCurrentCamera.vi"("error in (no error)"=w250, "cameraHandle"=w251) -> ("error out"=w248:errorcluster)  [unwired: 1 out]
                            n428 = call <userlib>:"SetTemperature.vi"("error in (no error)"=w248, "temperature"=w247) -> ("error out"=w249:errorcluster)  [unwired: 1 out]
                            n429 = call <userlib>:"CoolerON.vi"("error in (no error)"=w249) -> ()  [unwired: 1 in, 2 out]
                          }
                          frame "Cooling" {
                            n430 = call <userlib>:"GetCameraHandle.vi"("cameraIndex"=0) -> ("error out"=w258:errorcluster, "cameraHandle"=w259:i32)  [unwired: 2 in, 1 out]
                            n431 = call <userlib>:"SetCurrentCamera.vi"("error in (no error)"=w258, "cameraHandle"=w259) -> ("error out"=w257:errorcluster)  [unwired: 1 out]
                            n432 = call <userlib>:"SetTemperature.vi"("error in (no error)"=w257, "temperature"=w255) -> ("error out"=w261:errorcluster)  [unwired: 1 out]
                            n433 = call <userlib>:"GetTemperature.vi"("error in (no error)"=w261) -> ("status"=w262:T16, "temperature"=→"Current T(°C)":i32)  [unwired: 3 in, 2 out]
                            n434 = Not Equal?(x=w262, y=u32 36) -> (x != y?=→"Cooling":bool)
                          }
                        }
                      }
                      frame True {
                      }
                    }
                  }
                  frame #1 {
                    n435 = case shown="False" w267 {
                      tunnel: w266 -> [w270 _]
                      tunnel: [w269 _] -> w265
                      tunnel: w264 -> [w268 _]
                      frame False {
                        n436 = case shown="\"Cooling\"" w268 {
                          tunnel: w270 -> [w272 w279]
                          tunnel: [enum16{"Start Cooling", "Cooling"}."Cooling" enum16{"Start Cooling", "Cooling"}."Cooling"] -> w269
                          frame "Start Cooling" {
                            n437 = call <userlib>:"GetCameraHandle.vi"("cameraIndex"=1) -> ("error out"=w274:errorcluster, "cameraHandle"=w275:i32)  [unwired: 2 in, 1 out]
                            n438 = call <userlib>:"SetCurrentCamera.vi"("error in (no error)"=w274, "cameraHandle"=w275) -> ("error out"=w273:errorcluster)  [unwired: 1 out]
                            n439 = call <userlib>:"SetTemperature.vi"("error in (no error)"=w273, "temperature"=w272) -> ("error out"=w277:errorcluster)  [unwired: 1 out]
                            n440 = call <userlib>:"CoolerON.vi"("error in (no error)"=w277) -> ()  [unwired: 1 in, 2 out]
                          }
                          frame "Cooling" {
                            n441 = call <userlib>:"GetCameraHandle.vi"("cameraIndex"=1) -> ("error out"=w282:errorcluster, "cameraHandle"=w283:i32)  [unwired: 2 in, 1 out]
                            n442 = call <userlib>:"SetCurrentCamera.vi"("error in (no error)"=w282, "cameraHandle"=w283) -> ("error out"=w281:errorcluster)  [unwired: 1 out]
                            n443 = call <userlib>:"SetTemperature.vi"("error in (no error)"=w281, "temperature"=w279) -> ("error out"=w285:errorcluster)  [unwired: 1 out]
                            n444 = call <userlib>:"GetTemperature.vi"("error in (no error)"=w285) -> ("status"=w286:T16, "temperature"=→"Current T(°C) 2":i32)  [unwired: 3 in, 2 out]
                            n445 = Not Equal?(x=w286, y=u32 36) -> (x != y?=→"Cooling 2":bool)
                          }
                        }
                      }
                      frame True {
                      }
                    }
                  }
                }
              }
            }
          }
          event "Start": Value Change {
            n446 = event-data() -> ()  [unwired: 1 in, 6 out]
          }
          event "Stop": Value Change {
            n447 = event-data() -> ()  [unwired: 1 in, 6 out]
          }
          event "Quit Program": Value Change {
            w291 = FALSE ("Start Cooling")
            n448 = event-data() -> ("NewVal"=w292:bool)  [unwired: 1 in, 5 out]
            n449 = local write "Cooling On"(w291) -> ()
            n450 = local write "Cooling"(w291) -> ()
            n451 = local write "Cooling 2"(w291) -> ()
          }
          event "System Shut Down": Value Change {
            w293 = FALSE ("Start Cooling")
            n452 = event-data() -> ("NewVal"=w294:bool)  [unwired: 1 in, 5 out]
            n453 = local write "Cooling On"(w293) -> ()
            n454 = local write "Cooling"(w293) -> ()
            n455 = local write "Cooling 2"(w293) -> ()
          }
        }
      }
    }
  }
  "error out" <- w8
